vi "Main Traction Receipe Run.vi"(8 "error in (no error)":errorcluster, 11 "main ref":T1) -> (0 "error out":errorcluster)   [LabVIEW 2025]
uses:
  Traction Receipe Enum.ctl
  controls/LAB-IQ UI Data.ctl
panel:
  in  "Enum - Menu":T2
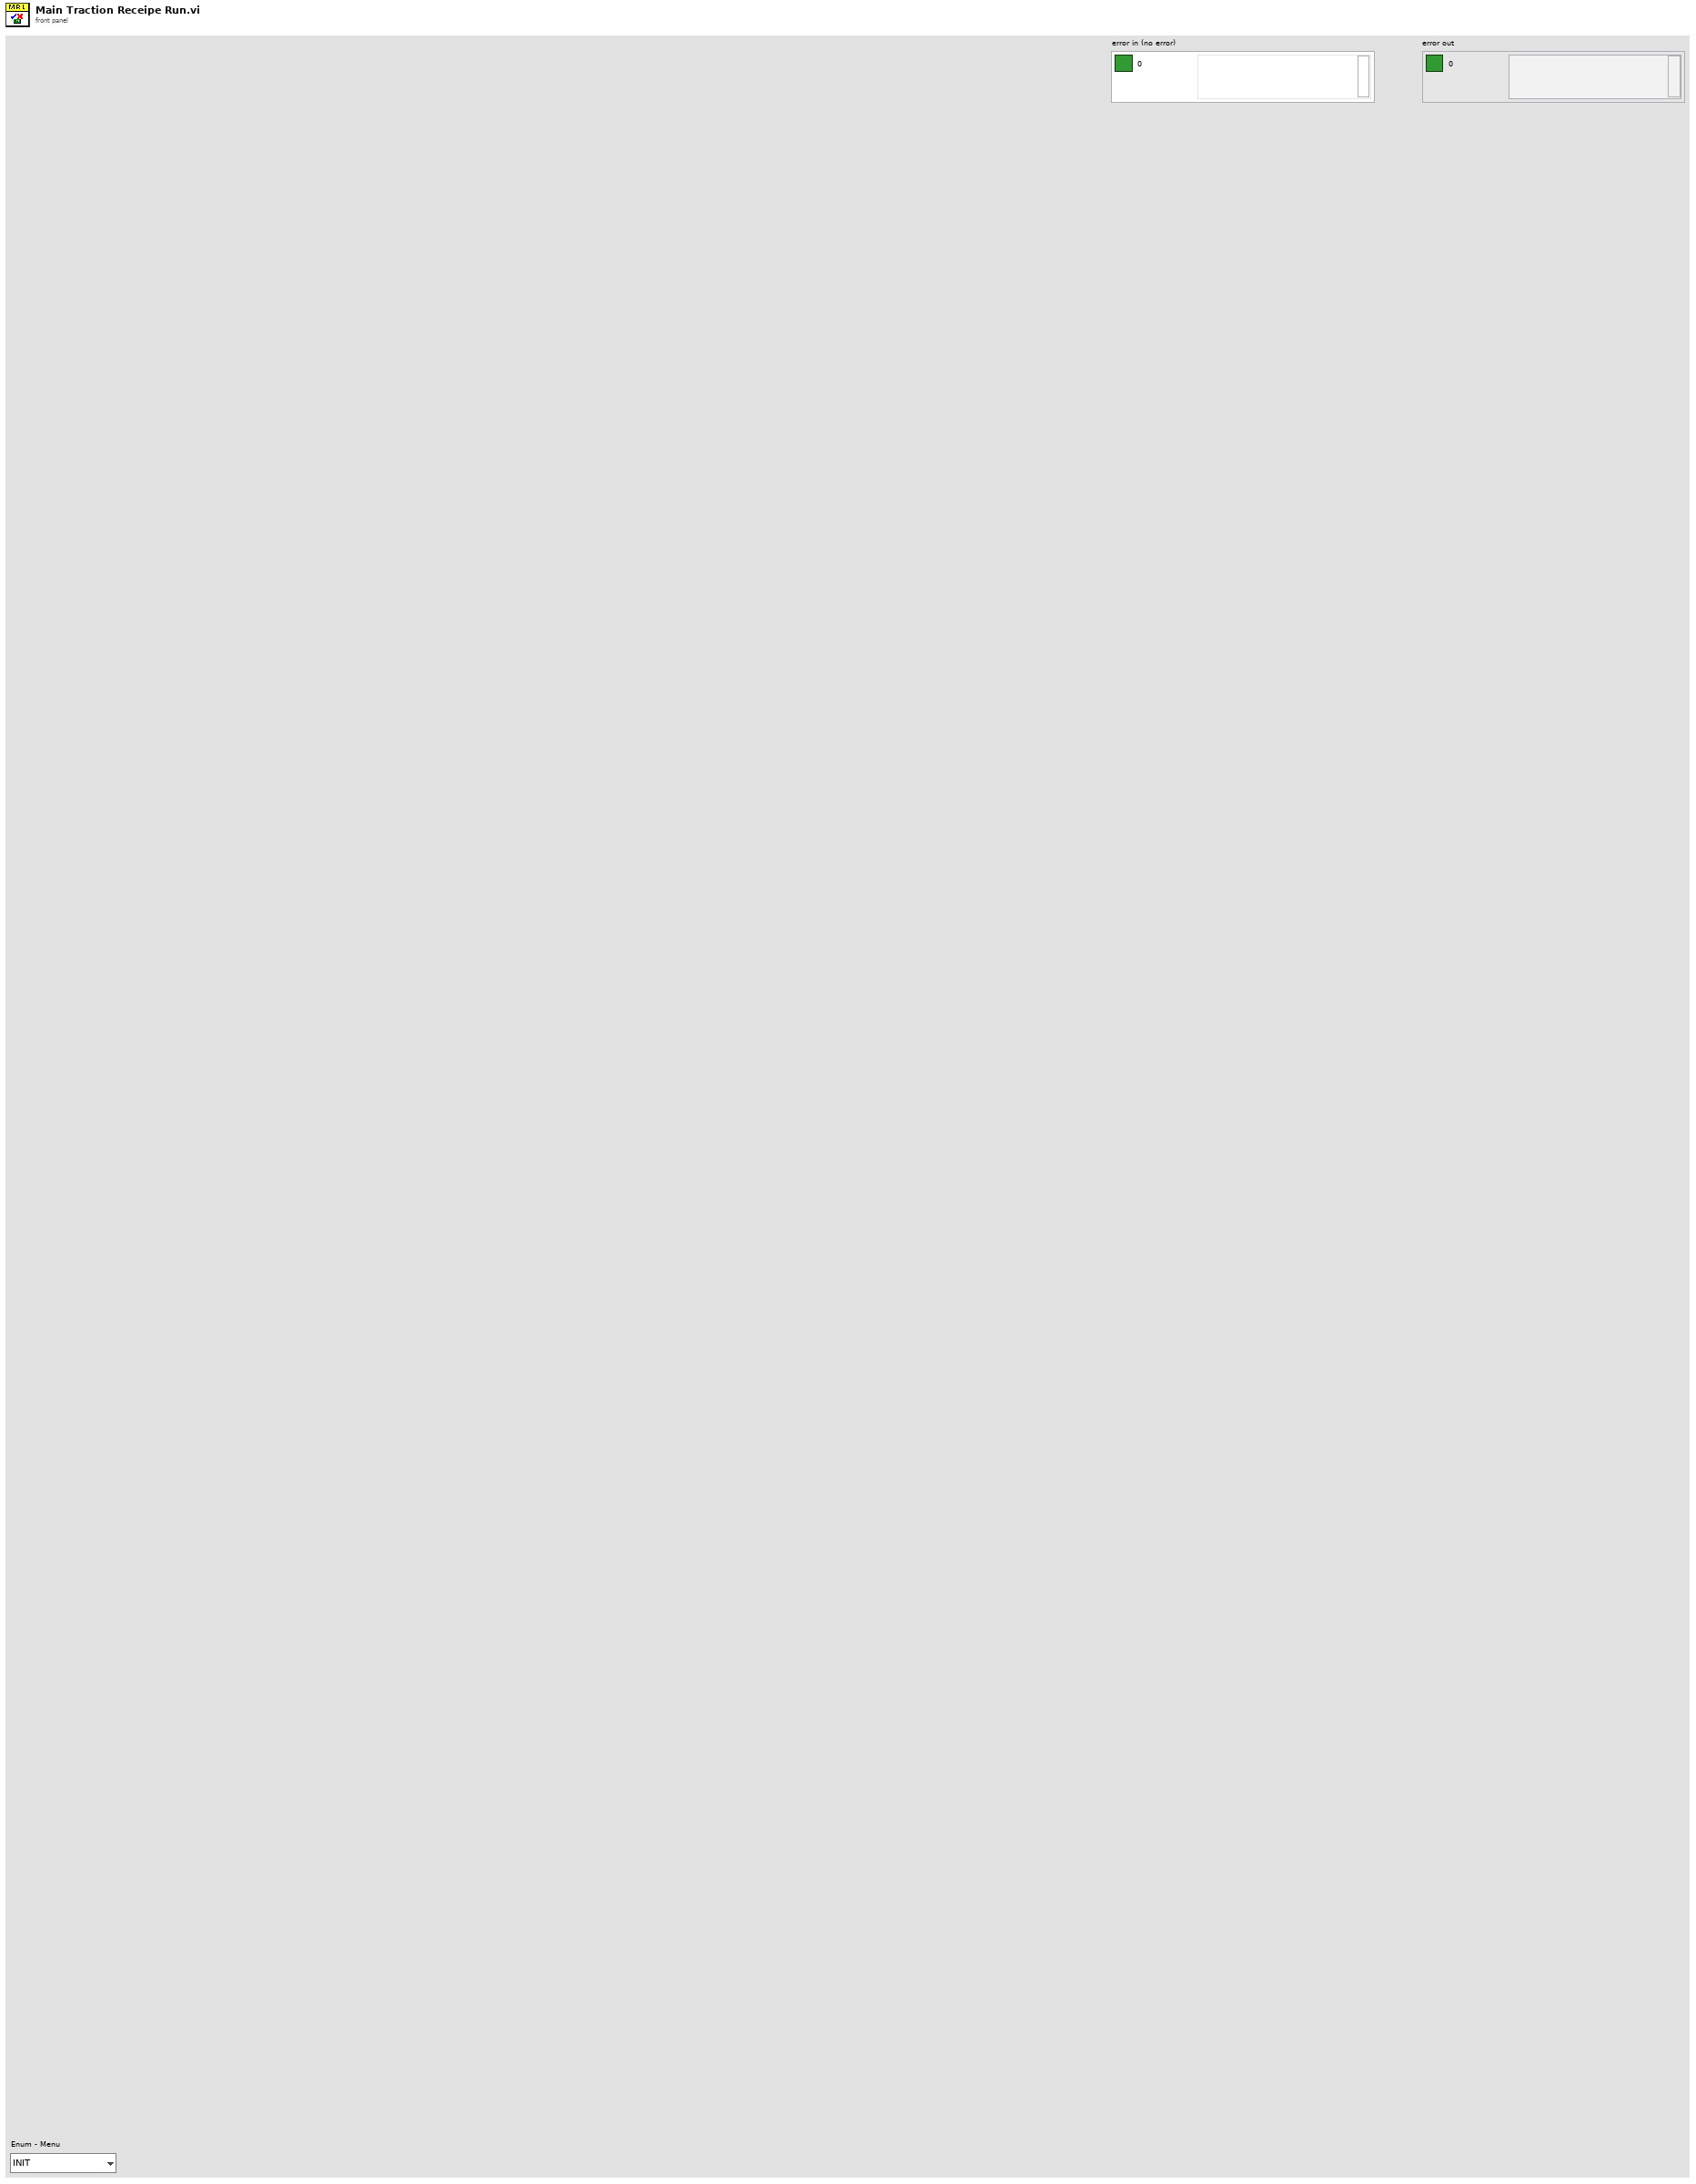
[diagram p1: front panel]
types:
  T1 = typedef "LAB-IQ UI Data.ctl" = cluster{"Main Home Screen":cluster{"GUI":refnum<vi>, "Platform Settings":refnum<vi>, "Configure":refnum<vi>, "Home":refnum<vi>, "EXIT":refnum<vi>, "service 2":refnum<vi>, "MainPage":refnum<vi>, "Analysis":refnum<vi>}, "Platform Settings":cluster{"mm/s  Surge":refnum<vi>, "Update Surge Speed":refnum<vi>, "Drive Error":refnum<vi>, "Disable Axis Jog Soft Limits":refnum<vi>, "mm/s  Sway":refnum<vi>, "Sway and Surge COM Status":refnum<vi>, "Heave COM Status":refnum<vi>, "Enable Platform":refnum<vi>, "Surge Forward Main":refnum<vi>, "Sway Right Main":refnum<vi>, "Sway Left Main":refnum<vi>, "Heave Down Main":refnum<vi>, "Heave Up main":refnum<vi>, "Update Sway Speed":refnum<vi>, "Update Heave Speed":refnum<vi>, "mm/s Heave":refnum<vi>, "mm/sec":refnum<vi>, "mm":refnum<vi>, "Surge Backward Main":refnum<vi>}, "Analysis Screen":cluster{"Analysis Home":refnum<vi>, "Surface Analysis":refnum<vi>, "Imaging":refnum<vi>, "Image Analysis":refnum<vi>, "Post Analysis":refnum<vi>}, "Config Screen":cluster{"Select Load Head":refnum<vi>, "Notes :":refnum<vi>, "FILE":refnum<vi>, "Sample ID :":refnum<vi>, "Operator ID :":refnum<vi>, "Operator Name :":refnum<vi>, "Auto":refnum<vi>}, "Motion Module":cluster{"zNL":refnum<vi>, "NL disp":refnum<vi>, "Rotary Tab":refnum<vi>, "Motion Direction:  3":refnum<vi>, "E.Velocity 2":refnum<vi>, "e.v/ssr 2":refnum<vi>, "Enter Fixed E.Velocity 2":refnum<vi>, "Enter Final SRR 2":refnum<vi>, "Enter initial SRR 2":refnum<vi>, "Enter Fixed SRR 2":refnum<vi>, "Enter the Final E.Velocity (m/s) 2":refnum<vi>, "Enter initial E.Velocity (m/s) 2":refnum<vi>, "Final Speed (RPM) 3":refnum<vi>, "Initial Speed (RPM) 2":refnum<vi>, "Enter the Final Velocity (m/s) 3":refnum<vi>, "Enter initial Velocity (m/s)  3":refnum<vi>, "Ramp Up 2":refnum<vi>, "TEST SELECTION":refnum<vi>, "SPEED SELECTION : ":refnum<vi>, "Angular Oscillation Set":refnum<vi>, "Traction":refnum<vi>, "Step Speed":refnum<vi>, "StepTable For Load-Speed":refnum<vi>, "StepTable For Speed":refnum<vi>, "Surge Forward MM":refnum<vi>, "Surge Backward MM":refnum<vi>, "M3 Image":refnum<vi>, "String 39":refnum<vi>, "Sway Left MM":refnum<vi>, "Sway Right MM":refnum<vi>, "Disable Axis Jog Soft Limits":refnum<vi>, "mm":refnum<vi>, "Heave Down MM":refnum<vi>, "Heave Up MM":refnum<vi>, "Wear Track Diameter (mm)":refnum<vi>, "Set WTD":refnum<vi>, "HomeScratch":refnum<vi>, "HomeRot":refnum<vi>, "PlaceModule":refnum<vi>, "Enter the Angle (Deg)":refnum<vi>, "Enter the Frequency (Hz)":refnum<vi>, "Motion Mode:":refnum<vi>, "LR Sway":refnum<vi>, "Rot Hor":refnum<vi>, "Scratch":refnum<vi>, "LR Cam":refnum<vi>, "MMBack":refnum<vi>, "MMNext":refnum<vi>, "Rot Ver":refnum<vi>, "Rotary Module Selection":refnum<vi>, "calculate rotary":refnum<vi>, "SPEED SELECTION : rotary":refnum<vi>, "Import 2":refnum<vi>, "Save 2":refnum<vi>, "File Path :  2":refnum<vi>, "String 45":refnum<vi>, "StepTable For Speed 3":refnum<vi>, "Enter the Speed(mm/sec)":refnum<vi>, "Enter the Speed(RPM)":refnum<vi>, "Enter Scratch Speed (mm/s):":refnum<vi>, "SwaySpeed Set":refnum<vi>, "Scartch Offset":refnum<vi>, "Motion type:":refnum<vi>, "HomeScratch 2":refnum<vi>, "Enter Scratch length (mm):":refnum<vi>, "Wear Track Diameter":refnum<vi>, "Rotary Speed Exced":refnum<vi>, "Scratch Mode":refnum<vi>, "No of Scratch":refnum<vi>}, "Environmental control":cluster{"Humidity  Status  3":refnum<vi>, "Low Temp  Status  2":refnum<vi>, "TK4 status 2":refnum<vi>, "Stage Temperature":refnum<vi>, "Sample Temperature":refnum<vi>, "Humidity (Amb)":refnum<vi>, "Clear List":refnum<vi>, "Add to list":refnum<vi>, "Wear":refnum<vi>, "Vibration":refnum<vi>, "Humidity (Chamber)":refnum<vi>, "Temperature (Chamber)":refnum<vi>, "ECR ":refnum<vi>, "Temperature (Amb)":refnum<vi>, "Microphone":refnum<vi>, "Acoustic Emission 3":refnum<vi>, "SNext":refnum<vi>, "APBack":refnum<vi>, "Enter the Temperature (°C):":refnum<vi>, "Enter the Stage \nTemperature (°C):":refnum<vi>, "Enter the Humidity (%Rh):":refnum<vi>, "Low Temp":refnum<vi>, "High Temp":refnum<vi>, "Humidity":refnum<vi>, "Sensors Picked":refnum<vi>}, "About Screen":cluster{"Password":refnum<vi>, "Home Service":refnum<vi>, "Advanced Setting":refnum<vi>, "About Tab":refnum<vi>, "ECR Port:":refnum<vi>, "Ramp Port:":refnum<vi>, "Installation/Replacement completed":refnum<vi>, "Loahead":refnum<vi>, "Heave and Surge COM Port:":refnum<vi>, "Sway COM Port:":refnum<vi>, "Temp Modbus:":refnum<vi>, "Humidity Port:":refnum<vi>, "Edit Gain Constants":refnum<vi>, "Save Gain Constants":refnum<vi>}, "Main Screen":cluster{"Main Screen Tab":refnum<vi>, "Angle and Frequency":refnum<vi>, "Stroke (mm)":refnum<vi>, "Angle (Deg)":refnum<vi>, "Main Speed Tab":refnum<vi>, "MTM MOTOR DISPLAY":refnum<vi>, "Disc Speed (m/sec)":refnum<vi>, "Ball Speed (m/sec)":refnum<vi>, "Disc Speed (RPM)":refnum<vi>, "Ball Speed (RPM)":refnum<vi>, "SPEED TAB":refnum<vi>, "Speed (m/sec)":refnum<vi>, "Set Speed (m/sec)":refnum<vi>, "Speed (RPM)":refnum<vi>, "Set Speed":refnum<vi>, "Time Tab":refnum<vi>, "Time ( HH:MM:SS ) 2":refnum<vi>, "Test Duration":refnum<vi>, "Test Duration 4":refnum<vi>, "TEST CYCLE":refnum<vi>, "TOTAL CYCLES":refnum<vi>, "Set Load (N)":refnum<vi>, "Temp Tabs":refnum<vi>, "Heater":refnum<vi>, "TK4 status":refnum<vi>, "ChamberTemp":refnum<vi>, "SetTmp":refnum<vi>, "Controller  Status":refnum<vi>, "ChamberTemp 2":refnum<vi>, "SetTmp 2":refnum<vi>, "Controller  Status 2":refnum<vi>, "ChamberTemp 3":refnum<vi>, "SetTmp 3":refnum<vi>, "Cooling":refnum<vi>, "Load Communication":refnum<vi>, "Ambient \nTemperature":refnum<vi>, "HumCOMStatus":refnum<vi>, "Ambient\n Humidity":refnum<vi>, "Freq (Hz)":refnum<vi>, "Load En":refnum<vi>, "NLt":refnum<vi>, "zNL 2":refnum<vi>, "Humidity On":refnum<vi>, "humidity disp":refnum<vi>, "Set Humidity":refnum<vi>, "NL disp 2":refnum<vi>, "Humidity On 2":refnum<vi>, "humidity disp 2":refnum<vi>, "Set Humidity 2":refnum<vi>, "NL disp 3":refnum<vi>, "AppLoadSeq scratch":refnum<vi>, "Stop Scratch":refnum<vi>, "ClrLog":refnum<vi>, "Trip Log":refnum<vi>, "STOP":refnum<vi>, "Start Test":refnum<vi>, "Test status":refnum<vi>, "AR Led":refnum<vi>, "Data":refnum<vi>, "Health":refnum<vi>, "Sway COM Status":refnum<vi>, "Heave COM Status":refnum<vi>, "Grp Tab":refnum<vi>, "Sub Graph":refnum<vi>, "SD (mm)":refnum<vi>, "Siliding distance Reset Graph":refnum<vi>, "SDGp":refnum<vi>, "Humidity Reset Graph":refnum<vi>, "HumrGp":refnum<vi>, "Acoustic Emission (mV)":refnum<vi>, "Aqucostic Reset Graph":refnum<vi>, "gACQUOS":refnum<vi>, "ECR RESET":refnum<vi>, "ECR":refnum<vi>, "Temperature Reset":refnum<vi>, "Acoustic Emission (mV) 2":refnum<vi>, "Aqucostic Reset Graph 2":refnum<vi>, "gACQUOS 2":refnum<vi>, "ECR RESET 2":refnum<vi>, "ECR 2":refnum<vi>, "Temperature Reset 2":refnum<vi>, "Temperature (deg c)":refnum<vi>, "Speed Reset Graph":refnum<vi>, "Speed Tab":refnum<vi>, "MTM DISC  SPEED":refnum<vi>, "MTM BALL SPEED":refnum<vi>, "speed mm/sec":refnum<vi>, "Hymidity":refnum<vi>, "Humidity Disable trip":refnum<vi>, "CoF Trip  2":refnum<vi>, "Depth Trip":refnum<vi>, "Weart Deapth":refnum<vi>, "Depth Reset Graph":refnum<vi>, "Weart":refnum<vi>, "Depthz":refnum<vi>, "Depth (µm)":refnum<vi>, "WearGp":refnum<vi>, "NL Trip 2":refnum<vi>, "Load pid":refnum<vi>, "Load Disable Trip":refnum<vi>, "Load Reset Graph":refnum<vi>, "NL Display 4":refnum<vi>, "Main Chart 3":refnum<vi>, "BACK":refnum<vi>, "Depth Trip 2":refnum<vi>, "COF TRIP ":refnum<vi>, "Friction Force (N)":refnum<vi>, "FF Reset Graph":refnum<vi>, "FF Disable Trip":refnum<vi>, "FF TRIP":refnum<vi>, "COF Disable Trip":refnum<vi>, "COF Reset Graph":refnum<vi>, "Start Test Temp":refnum<vi>, "zFF":refnum<vi>, "Friction Force (N) Graph":refnum<vi>, "Coefficient of Friction":refnum<vi>, "Scratch Start Test":refnum<vi>, "FF Tab":refnum<vi>, "Cyclic Friction Force (N)":refnum<vi>, "CZ FF":refnum<vi>, "Cyclic Friction Force (N) Graph":refnum<vi>, "Cyclic Coefficient of Friction":refnum<vi>, "Cyclic FF TRIP":refnum<vi>, "Cyclic FF Disable Trip":refnum<vi>, "cyclic COF Disable Trip":refnum<vi>, "cyclic COF TRIP":refnum<vi>, "cyclic COF Reset Graph":refnum<vi>, "Cyclic FF Reset Graph":refnum<vi>, "Test Trip":refnum<vi>, "Multi Scratch Pass":refnum<vi>, "Scratch Start Recording":refnum<vi>}, "Loading":cluster{"Indentation":refnum<vi>, "Reference Sample":refnum<vi>, "Load Cell Communication Slide":refnum<vi>, "com 3":refnum<vi>, "com":refnum<vi>, "DecaForce COM Status":refnum<vi>, "Update":refnum<vi>, "Clear 3":refnum<vi>, "seq":refnum<vi>, "Stribeck table":refnum<vi>, "Stribeck Table  For loading":refnum<vi>, "Loading Mode":refnum<vi>, "Enter the Final Load (N)":refnum<vi>, "Enter the CoF Trip":refnum<vi>, "Enter the Friction Force Trip":refnum<vi>, "Enter the Normal load Trip":refnum<vi>, "Enter the Load  (N)":refnum<vi>, "KiloForce":refnum<vi>, "DecaForce ":refnum<vi>, "MicroForce":refnum<vi>, "LHBack":refnum<vi>, "LHNext":refnum<vi>, "Enter the Loading Rate (N/min)":refnum<vi>, "Message":refnum<vi>, "Warning 2":refnum<vi>, "SSP 0.75":refnum<vi>, "SSP 0.5":refnum<vi>, "SSP 0.3":refnum<vi>, "Warning":refnum<vi>, "gui GIF":refnum<vi>, "Communication is established":refnum<vi>, "AppLoad 4":refnum<vi>, "Multipoint":refnum<vi>, "Load Selection":refnum<vi>}, "PID":cluster{"Ramp MulFac":refnum<vi>, "pulses LoadDiffRamp(2..10)":refnum<vi>, "PulseControlRamp(diff<=3N)":refnum<vi>, "SetLoadDeadband(%) Load(0-10N)":refnum<vi>, "PID gains out delay (microForce)":refnum<vi>, "Ramp":refnum<vi>, "Gain 2":refnum<vi>, "pulses LoadDiff(2..10)":refnum<vi>, "pulses LoadDiff(11..50)":refnum<vi>, "PulseControl(diff<=3N)":refnum<vi>, "SetLoadDeadband(%)  2":refnum<vi>, "Dummy Run":refnum<vi>, "Vertical load (N)":refnum<vi>, "AutoTune":refnum<vi>, "Offset 3 ":refnum<vi>, "apply load":refnum<vi>, "Offset  3":refnum<vi>, "apply load 2":refnum<vi>, "Enter ByPass Load":refnum<vi>, "reinit 3":refnum<vi>, "output range delay":refnum<vi>, "PID gains out delay":refnum<vi>, "Bypass Load":refnum<vi>, "pulsesSent":refnum<vi>, "pulses ":refnum<vi>, "actpid":refnum<vi>, "gFF Rot":refnum<vi>, "pulses LoadDiff(21..1000)":refnum<vi>, "Delay":refnum<vi>, "deadband":refnum<vi>}, "Config Parameters":cluster{"Tab Control 3":refnum<vi>, "Tab Control 19":refnum<vi>, "SAMPLES":refnum<vi>, "Re-initilaize":refnum<vi>, "Filter ON/OFF":refnum<vi>, "TracHomeSurgeOffsetCounts 10MM":refnum<vi>, "TracHomeSwayOffsetCounts 10MM":refnum<vi>, "Acoustic Emission:":refnum<vi>, "Apply Filter (FF)":refnum<vi>, "Filter% 2":refnum<vi>, "Apply Filter (Load)":refnum<vi>, "Filter% ":refnum<vi>, "Sway distance (mm)":refnum<vi>, "Surge distance (mm)":refnum<vi>, "DataSavingLoopDelay(ms)":refnum<vi>, "SAVE 2":refnum<vi>, "Enter Distance":refnum<vi>, "Sway Counts:":refnum<vi>, "Distance (mm): 3":refnum<vi>, "Surge Counts:":refnum<vi>, "Distance (mm): 2":refnum<vi>, "Distance (mm):":refnum<vi>, "Heave Counts:":refnum<vi>, "LRMHomeSurgeOffsetCounts":refnum<vi>, "LRMHomeSwayOffsetCounts":refnum<vi>, "TracHomeSurgeOffsetCounts 20MM":refnum<vi>, "TracHomeSwayOffsetCounts 20MM":refnum<vi>, "RotHomeSwayOffsetCounts":refnum<vi>, "RotHomeSurgeOffsetCounts":refnum<vi>, "Heave distance":refnum<vi>, "Zmm":refnum<vi>, "Heave Pulses/mm":refnum<vi>, "Surge Pulses/mm":refnum<vi>, "Sway Pulses/mm":refnum<vi>, "Heave Pitch":refnum<vi>, "Surge Pitch":refnum<vi>, "Sway Pitch":refnum<vi>, "Heave PPR":refnum<vi>, "Surge PPR":refnum<vi>, "Sway PPR":refnum<vi>, "Tab Control 5":refnum<vi>, "Tab Control 14":refnum<vi>, "Tab Control 26":refnum<vi>, "AE":refnum<vi>, "Heave Loop Delay":refnum<vi>, "Heave PID Speed":refnum<vi>, "Surge Jog Speed":refnum<vi>, "Heave Jog Speed":refnum<vi>, "Sway Loop Delay":refnum<vi>, "Sway PID Speed":refnum<vi>, "Sway Jog Speed":refnum<vi>, "DEPTH TRIP VALUE":refnum<vi>, "LOAD TRIP VALUE":refnum<vi>, "DEPTH TRIP   ENABLE":refnum<vi>, "LOAD TRIP  ENABLE":refnum<vi>, "CYCLIC FF TRIP VALUE":refnum<vi>, "FF TRIP VALUE":refnum<vi>, "CYCLIC CoF TRIP VALUE":refnum<vi>, "COF TRIP VALUE":refnum<vi>, "CYCLIC COF TRIP  ENABLE":refnum<vi>, "CYCLIC FF TRIP  ENABLE":refnum<vi>, "FF TRIP  ENABLE":refnum<vi>, "COF TRIP  ENABLE":refnum<vi>, "JOG TRIP LOAD VALUE (N)":refnum<vi>, "Rotary Vertical":refnum<vi>, "Traction":refnum<vi>, "Scratch":refnum<vi>, "LRM CAM":refnum<vi>, "Sway LRM":refnum<vi>, "Rotary Horizontal":refnum<vi>}, "Loading Com Port":cluster{"ClearAll":refnum<vi>, "Mz(Nm)":refnum<vi>, "My(Nm)":refnum<vi>, "Mx(Nm)":refnum<vi>, "Save Dwell":refnum<vi>, "Acq Delay (ms)":refnum<vi>, "Burst Delay (ms)":refnum<vi>, "model":refnum<vi>, "SN":refnum<vi>, "FFx(N)":refnum<vi>, "Sensor IP":refnum<vi>, "Port":refnum<vi>, "FFy(N)":refnum<vi>, "Load(N)":refnum<vi>, "delete Handle":refnum<vi>, "Create Handle":refnum<vi>, "ft_data":refnum<vi>, "ft_range":refnum<vi>, "ft_data 2":refnum<vi>, "stop 6":refnum<vi>, "running_flag":refnum<vi>, "ft_udp_handle":refnum<vi>, "get-data-return":refnum<vi>, "get-range-return":refnum<vi>, "zero-return":refnum<vi>, "filter-return":refnum<vi>, "initial-return":refnum<vi>, "deleteHandle-result":refnum<vi>, "Load Cell Temp":refnum<vi>, "Load Cell":refnum<vi>, "ZeroAll":refnum<vi>, "FORCE (N)":refnum<vi>, "TORQUE (N-m)":refnum<vi>}, "Heave AND Surge":cluster{"SURGE POSE":refnum<vi>, "error out Read":refnum<vi>, "HEAVE POSE":refnum<vi>, "State":refnum<vi>, "Homed":refnum<vi>, "Sequence ID":refnum<vi>, "error out Write":refnum<vi>, "faultCode":refnum<vi>, "Ack ID":refnum<vi>, "SPEED":refnum<vi>, "Distance":refnum<vi>, "Mode Command":refnum<vi>, "Heave and Surge Read":refnum<vi>, "Read Heave Temp":refnum<vi>, "Spare 15":refnum<vi>, "Spare 14":refnum<vi>, "Spare 13":refnum<vi>, "Spare 12":refnum<vi>, "Spare 11":refnum<vi>, "Spare 10":refnum<vi>, "Spare 9":refnum<vi>, "Spare 8":refnum<vi>, "Spare 7":refnum<vi>, "Spare 6":refnum<vi>, "Spare 5":refnum<vi>, "Spare 4":refnum<vi>, "Spare 2":refnum<vi>, "Spare 1":refnum<vi>, "Node Id":refnum<vi>, "Spare 3":refnum<vi>, "SPARE 4":refnum<vi>, "SPARE 3":refnum<vi>, "SPARE 2":refnum<vi>, "SPARE 1":refnum<vi>, "fwMajor":refnum<vi>, "fwMinor":refnum<vi>, "Manual Write":refnum<vi>, "Heave and Surge Write":refnum<vi>, "SPARE 5":refnum<vi>, "Reserved ":refnum<vi>, "SPARE 8":refnum<vi>, "SPARE 6":refnum<vi>, "SPARE 7":refnum<vi>, "SPARE 17":refnum<vi>, "SPARE 16":refnum<vi>, "SPARE 15":refnum<vi>, "SPARE 14":refnum<vi>, "SPARE 13":refnum<vi>, "SPARE 12":refnum<vi>, "SPARE 11":refnum<vi>, "SPARE 10":refnum<vi>, "SPARE 9":refnum<vi>, "System UPTIME":refnum<vi>, "Missed Packets":refnum<vi>, "faultCode Surge Right":refnum<vi>, "faultCode Surge Left":refnum<vi>, "faultCode Heave":refnum<vi>, "UPLINK HEAVE":refnum<vi>, "DOWNLINK HEAVE":refnum<vi>}, "New PID LOGIC":cluster{"Fine Tune Zone":refnum<vi>, "PID SDelay":refnum<vi>, "Max_pos_limit":refnum<vi>, "Min_pos_limit":refnum<vi>, "i_limit":refnum<vi>, "pct_scale":refnum<vi>, "Deadband":refnum<vi>, "Kd":refnum<vi>, "Ki":refnum<vi>, "Kp":refnum<vi>, "Current Position":refnum<vi>, "Set Load":refnum<vi>, "Current Load":refnum<vi>, "Pulse delta":refnum<vi>, "Init Step":refnum<vi>, "Max Step Linit":refnum<vi>, "min_deadband_floor":refnum<vi>, "dynamic_spindle_noise_scalar":refnum<vi>, "min_finetune_floor":refnum<vi>, "filter_alpha":refnum<vi>, "PID":refnum<vi>}, "SWAY ":cluster{"fwMajor":refnum<vi>, "Homed":refnum<vi>, "Rotary POSE":refnum<vi>, "State":refnum<vi>, "SWAY POSE":refnum<vi>, "Ack ID":refnum<vi>, "faultCode":refnum<vi>, "Node Id":refnum<vi>, "fwMinor":refnum<vi>, "Spare 6":refnum<vi>, "Spare 5":refnum<vi>, "Spare 4":refnum<vi>, "Spare 3":refnum<vi>, "Spare 2":refnum<vi>, "Spare 1":refnum<vi>, "Spare 7":refnum<vi>, "SPARE  5":refnum<vi>, "error out Write  SWAY ":refnum<vi>, "error out Read SWAY ":refnum<vi>, "Manual Write SWAY ":refnum<vi>, "SWAY WRITE":refnum<vi>, "SPARE  4":refnum<vi>, "SPARE  3":refnum<vi>, "SPARE 2":refnum<vi>, "SPARE 1":refnum<vi>, "Spare 15":refnum<vi>, "Spare 14":refnum<vi>, "Spare 13":refnum<vi>, "Spare 12":refnum<vi>, "Spare 11":refnum<vi>, "Spare 9":refnum<vi>, "Spare 8":refnum<vi>, "SPEED":refnum<vi>, "Distance":refnum<vi>, "Mode Command":refnum<vi>, "Sequence ID":refnum<vi>, "SWAY READ":refnum<vi>, "Spare 10":refnum<vi>, "Read SWAY Temp":refnum<vi>, "faultCode Sway ":refnum<vi>, "Missed Packets":refnum<vi>, "System UPTIME sway":refnum<vi>, "SPARE 6":refnum<vi>, "SPARE 7":refnum<vi>, "SPARE 9":refnum<vi>, "SPARE 11":refnum<vi>, "SPARE 10":refnum<vi>, "SPARE 8":refnum<vi>, "SPARE 13":refnum<vi>, "SPARE 12":refnum<vi>, "SPARE 17":refnum<vi>, "SPARE 16":refnum<vi>, "SPARE 15":refnum<vi>, "SPARE 14":refnum<vi>, "Reserved":refnum<vi>, "faultCode Rotary":refnum<vi>, "UPLINK SWAY":refnum<vi>, "DOWNLINK SWAY":refnum<vi>}, "Analysis Screen":cluster{"Analysis Home":refnum<vi>, "Refresh 2":refnum<vi>, "MEAN 4":refnum<vi>, "SD 4":refnum<vi>, "VARIANCE 4":refnum<vi>, "MEAN  3":refnum<vi>, "SD  3":refnum<vi>, "VARIANCE  3":refnum<vi>, "MEAN 2":refnum<vi>, "SD  2":refnum<vi>, "VARIANCE 2":refnum<vi>, "MEAN":refnum<vi>, "SD":refnum<vi>, "VARIANCE":refnum<vi>, "File 4 Discription":refnum<vi>, "OPEN 4":refnum<vi>, "File Name 4":refnum<vi>, "OPEN 3":refnum<vi>, "File 3 Discription":refnum<vi>, "File Name 3":refnum<vi>, "Y-AXIS":refnum<vi>, "X-AXIS":refnum<vi>, "XY Graph":refnum<vi>, "File Name 2":refnum<vi>, "File Name 1":refnum<vi>, "OPEN 2":refnum<vi>, "OPEN 1":refnum<vi>, "File 1 Discription ":refnum<vi>, "File 2 Discription":refnum<vi>, "Export":refnum<vi>, "File Format":refnum<vi>}, "Traction":cluster{"faultCode Traction 2":refnum<vi>, "faultCode Traction 1":refnum<vi>, "Missed Packets":refnum<vi>, "System UPTIME Traction":refnum<vi>, "SPARE 17":refnum<vi>, "SPARE 16":refnum<vi>, "SPARE 15":refnum<vi>, "SPARE 14":refnum<vi>, "SPARE 13":refnum<vi>, "SPARE 12":refnum<vi>, "SPARE 11":refnum<vi>, "SPARE 10":refnum<vi>, "SPARE 9":refnum<vi>, "SPARE 8":refnum<vi>, "SPARE 7":refnum<vi>, "SPARE 6":refnum<vi>, "Reserved":refnum<vi>, "SPARE  5":refnum<vi>, "Manual Write TRACTION":refnum<vi>, "TRACTION WRITE":refnum<vi>, "SPARE  4":refnum<vi>, "SPARE  3":refnum<vi>, "SPARE 2":refnum<vi>, "SPARE 1":refnum<vi>, "Spare 7":refnum<vi>, "Spare 6":refnum<vi>, "Spare 5":refnum<vi>, "Spare 4":refnum<vi>, "Spare 2":refnum<vi>, "Spare 1":refnum<vi>, "Node Id":refnum<vi>, "Read TRACTION Temp":refnum<vi>, "fwMinor":refnum<vi>, "fwMajor":refnum<vi>, "faultCode":refnum<vi>, "TRACTION POSE":refnum<vi>, "TRACTION POSE 2":refnum<vi>, "Homed":refnum<vi>, "State":refnum<vi>, "Ack ID":refnum<vi>, "SPEED":refnum<vi>, "Distance":refnum<vi>, "Mode Command":refnum<vi>, "Sequence ID":refnum<vi>, "error out Read TRACTION":refnum<vi>, "error out Write  TRACTION":refnum<vi>, "TRACTION READ":refnum<vi>, "Spare 3":refnum<vi>, "Downlink traction":refnum<vi>, "Uplink Traction":refnum<vi>}, "Traction reciepe":cluster{"SRR Sweep Range (%) Stribeck":refnum<vi>, "Traction Receipe":refnum<vi>, "Total Execution Time":refnum<vi>, "Total Steps":refnum<vi>, "Duration / Step (s)  Stribeck":refnum<vi>, "STRIBECK Fixed SRR List (%)":refnum<vi>, "Duration / Step (s) Traction":refnum<vi>, "SRR Sweep Range (%) traction":refnum<vi>, "Rolling Speed (mm/s)":refnum<vi>, "Temperature Stages (°C)":refnum<vi>, "Ball Load (N)":refnum<vi>, "Lubricant Name":refnum<vi>, "Profile File Name":refnum<vi>, "SET entrainment Velocity":refnum<vi>, "Test Array Size":refnum<vi>, "SRR INDEX [ STRIBECK]":refnum<vi>, "Stribeck Size":refnum<vi>, "SET SRR":refnum<vi>, "ELAPSED TIMER ":refnum<vi>, "BALL SET RPM":refnum<vi>, "DISC SET RPM":refnum<vi>, "SET LOAD":refnum<vi>, "TEMPERATURE READ":refnum<vi>, "SET TEMPERATURE":refnum<vi>, "Traction Size":refnum<vi>, "DISC SPEED (rpm)":refnum<vi>, "BALL SPEED (rpm)":refnum<vi>, "BALL WEAR TRACK":refnum<vi>, "DISC WEARTRACK":refnum<vi>, "SRR INDEX [ TRACTION]":refnum<vi>, "Start Index Type":refnum<vi>, "Enum - Menu":refnum<vi>, "Ball (mm/sec)":refnum<vi>, "Disc (mm/sec)":refnum<vi>}, "Traction Control":cluster{"HomeTraction":refnum<vi>, "Demo Mode Display":refnum<vi>, "Traction Message":refnum<vi>, "Traction Step Update Details":refnum<vi>, "Main Tab sequence for selection":refnum<vi>, "Ramp Tab":refnum<vi>, "e.v/ssr":refnum<vi>, "Enter Fixed E.Velocity":refnum<vi>, "Enter Final SRR":refnum<vi>, "Enter initial SRR":refnum<vi>, "Enter Fixed SRR":refnum<vi>, "Enter the Final E.Velocity (m/s)":refnum<vi>, "Enter initial E.Velocity (m/s)":refnum<vi>, "Ball WTD":refnum<vi>, "E.Velocity":refnum<vi>, "Enter the Final Velocity (m/s)":refnum<vi>, "Enter initial Velocity (m/s)":refnum<vi>, "Ramp Up   Disc":refnum<vi>, "Initial DiscSpeed (RPM)":refnum<vi>, "Final Speed (RPM) Ball":refnum<vi>, "Final Speed (RPM)":refnum<vi>, "Initial Speed (RPM) Ball":refnum<vi>, "Enter the Final Velocity (m/s) Ball":refnum<vi>, "Enter initial Velocity (m/s) Ball":refnum<vi>, "Ramp Up":refnum<vi>, "ExceedBallSpeed step":refnum<vi>, "ExceedDiscSpeed":refnum<vi>, "BallSpeed Exceed Indication":refnum<vi>, "Apply":refnum<vi>, "SPEED SELECTION : MTM":refnum<vi>, "SPEED SELECTION : MTM 2":refnum<vi>, "TEST SELECTION (MTM)":refnum<vi>, "MTM Test Selection":refnum<vi>, "File Path Tab":refnum<vi>, "File Path String":refnum<vi>, "Save":refnum<vi>, "Save  2":refnum<vi>, "Import ":refnum<vi>, "File Path :":refnum<vi>, "Step Sequence Indication Tab":refnum<vi>, "Step Sequence Indication":refnum<vi>, "Calculate Step":refnum<vi>, "StepTable":refnum<vi>, "ExceedDiscSpeed  Cinstant Speed":refnum<vi>, "ExceedBallSpeed Constant":refnum<vi>, "TEST SELECTION (MTM) 2":refnum<vi>, "SPEED SELECTION : MTM 3":refnum<vi>, "MTM Test Selection 2":refnum<vi>, "Enter the Speed (m/sec): ":refnum<vi>, "Enter the Speed (m/sec):  2":refnum<vi>, "Enter the Speed (RPM):":refnum<vi>, "Lower Spped ":refnum<vi>, "Upper":refnum<vi>, "Enter the Speed (RPM):Ball":refnum<vi>, "Disc Motion Direction: ":refnum<vi>, "Ball Motion Direction :":refnum<vi>, "Motion Mode: ":refnum<vi>, "Wear Track Diameter (mm) ":refnum<vi>, "Disc Speed Indicator":refnum<vi>, "ExceedBallSpeed":refnum<vi>}, "Acquostic":cluster{"Last Config Rejected ":refnum<vi>, "rx command count":refnum<vi>, "Current Filter Id":refnum<vi>, "Isolated Gain":refnum<vi>, "DAQ Status":refnum<vi>, "error out":refnum<vi>, "error in (no error)":refnum<vi>, "Uplink Packet":refnum<vi>, "data out":refnum<vi>, "Downlink Packet":refnum<vi>, "Signal Energy":refnum<vi>, "Amplitude db_AE":refnum<vi>, "Peak Amplitude":refnum<vi>, "AE Ring-Down Counts":refnum<vi>, "Gains":refnum<vi>, "Manual Write Acquostic":refnum<vi>}}
  T2 = typedef "Traction Receipe Enum.ctl" = enum16{"INIT", "START", "TRACTION", "STRIBECK", "MAIN INDEX INCREMENT", "TEMPERATURE SET", "TEMPERATURE REACH", "CHURNING START", "CHURNING STOP", "LOAD", "LOAD REACHED", "SRR SET", "SRR WAIT", "SRR INCREMENT", "SPEED SET", "SPEED WAIT", "SPEED INCREMENT", "UNLOAD", "CLOSE"}
  T3 = enum8{"Enabled", "Disabled", "Disabled and Grayed Out"}
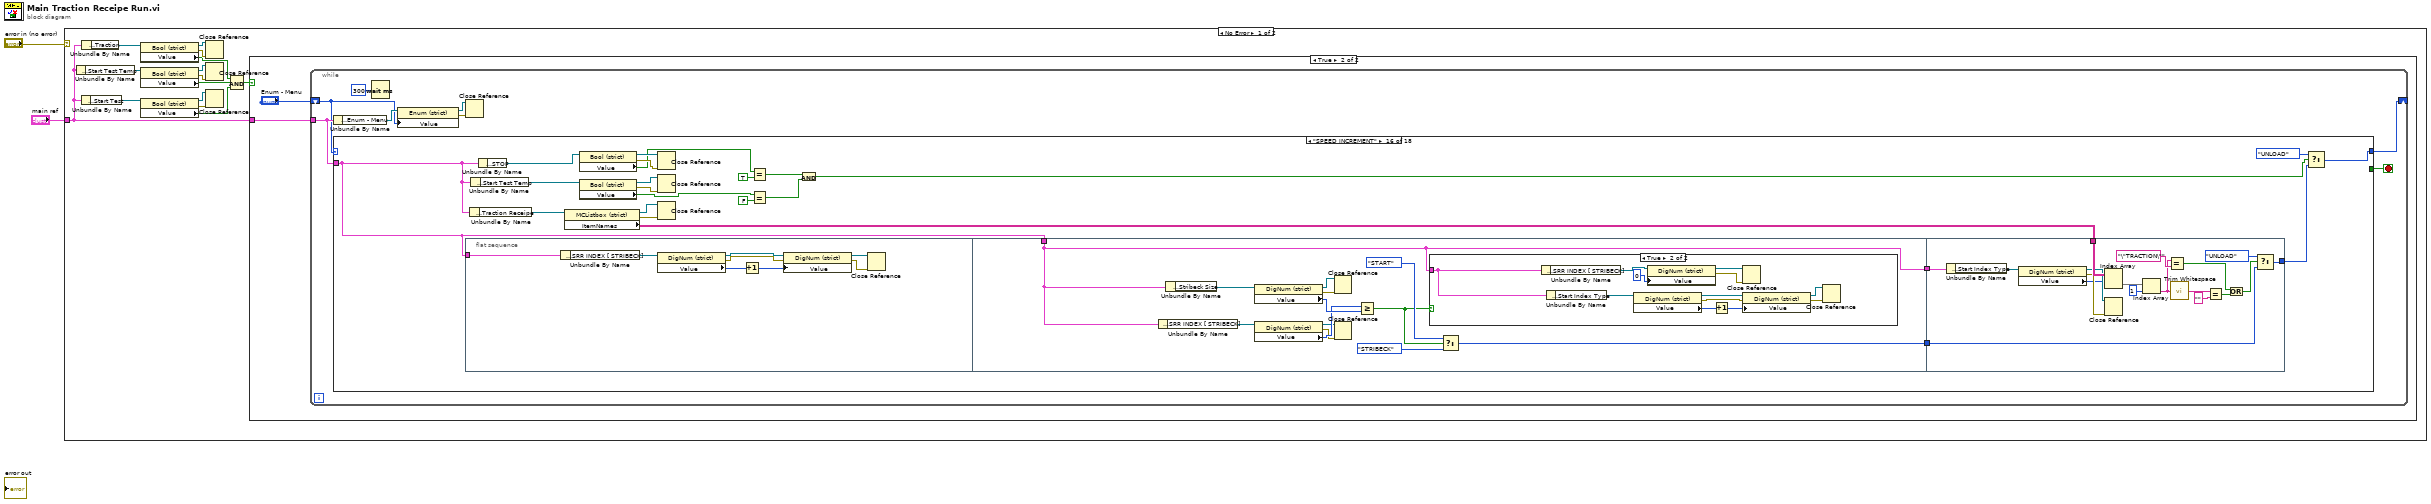
[diagram p0: block diagram]
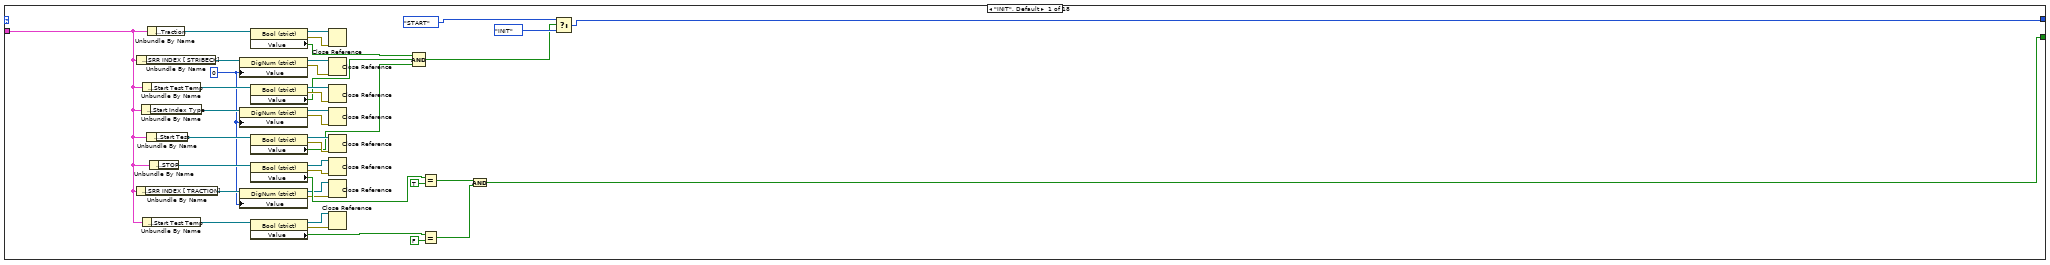
[diagram p3: hidden frame]
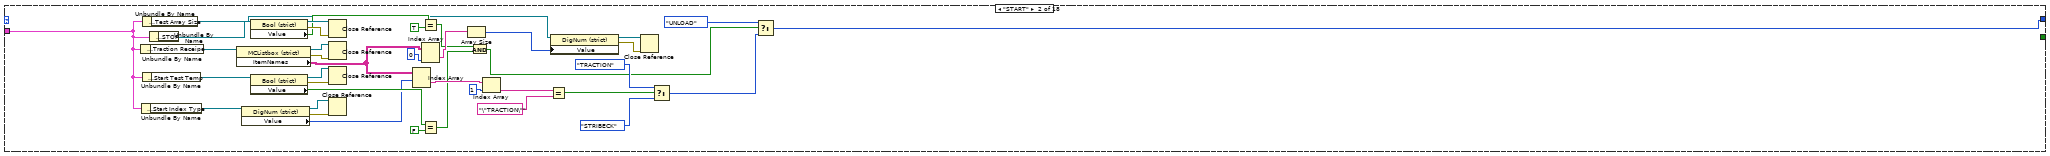
[diagram p4: hidden frame]
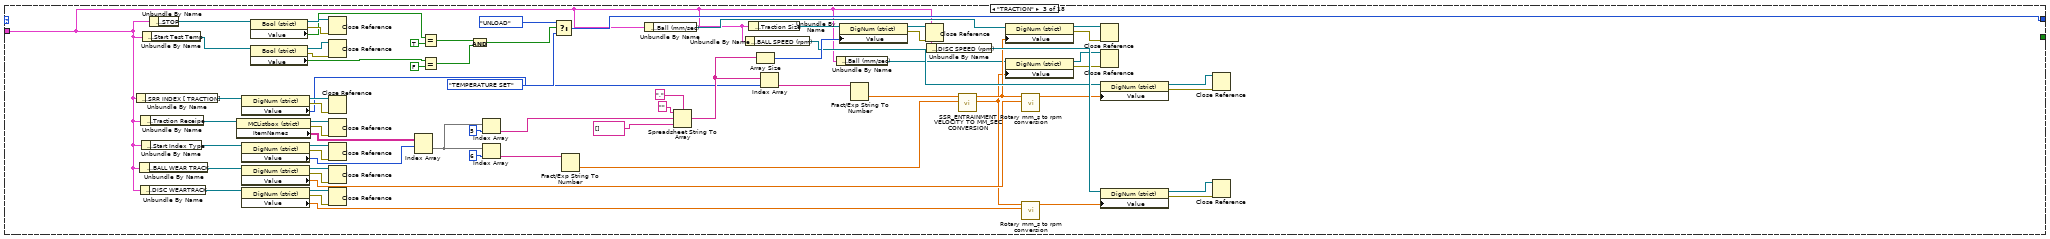
[diagram p5: hidden frame]
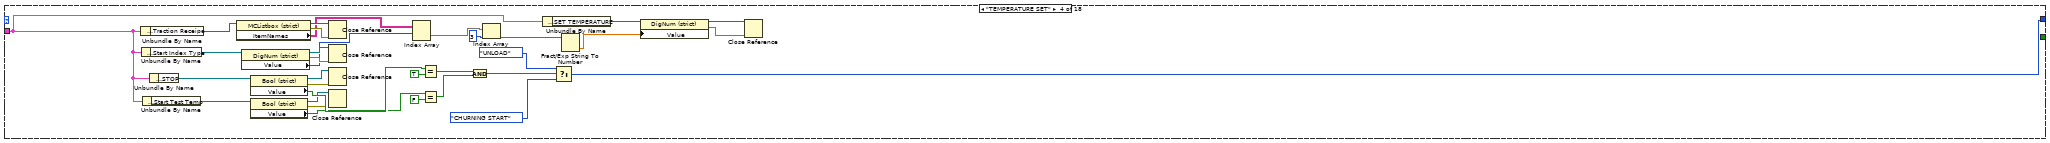
[diagram p6: hidden frame]
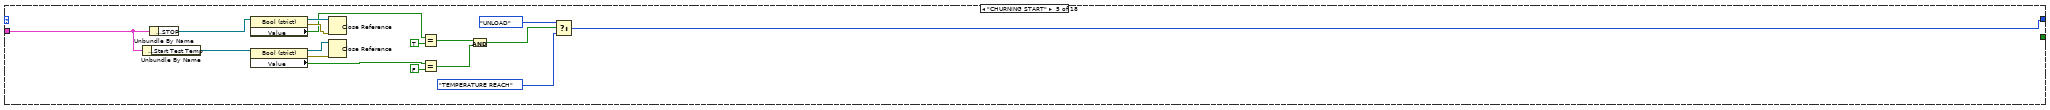
[diagram p7: hidden frame]
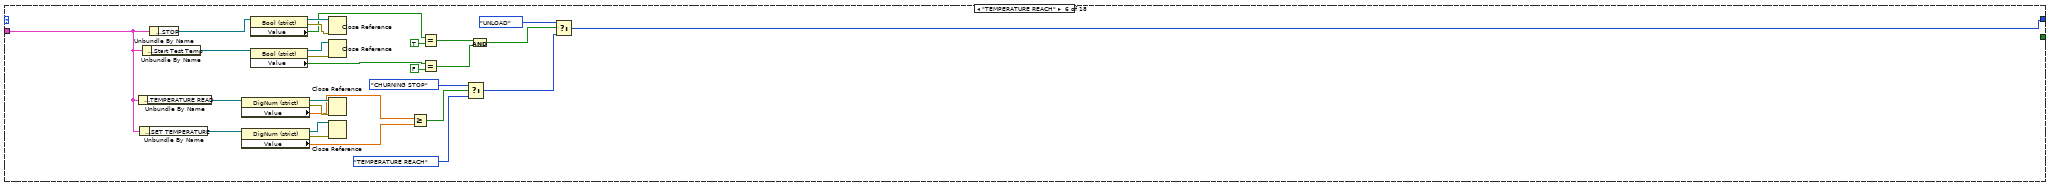
[diagram p8: hidden frame]
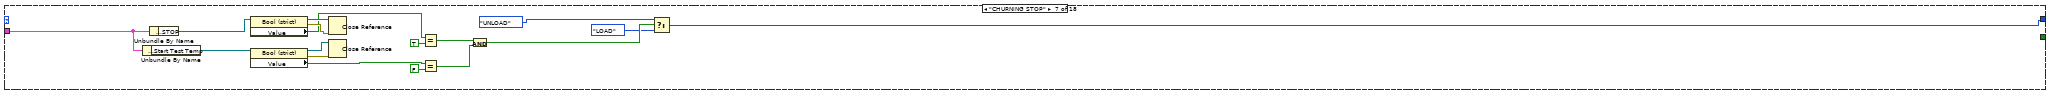
[diagram p9: hidden frame]
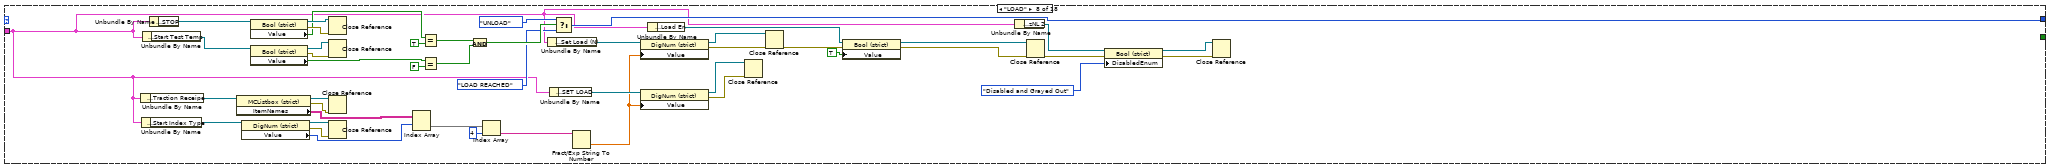
[diagram p10: hidden frame]
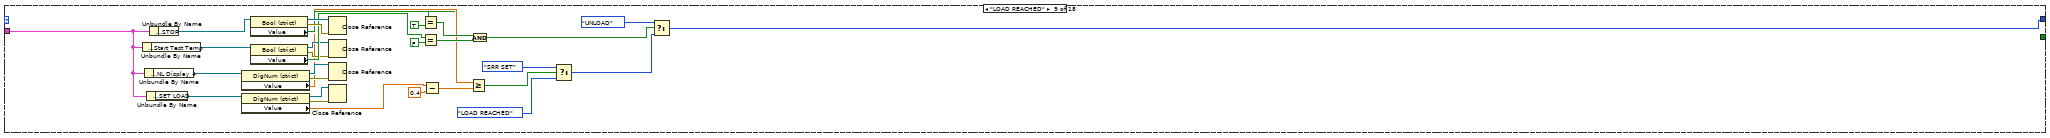
[diagram p11: hidden frame]
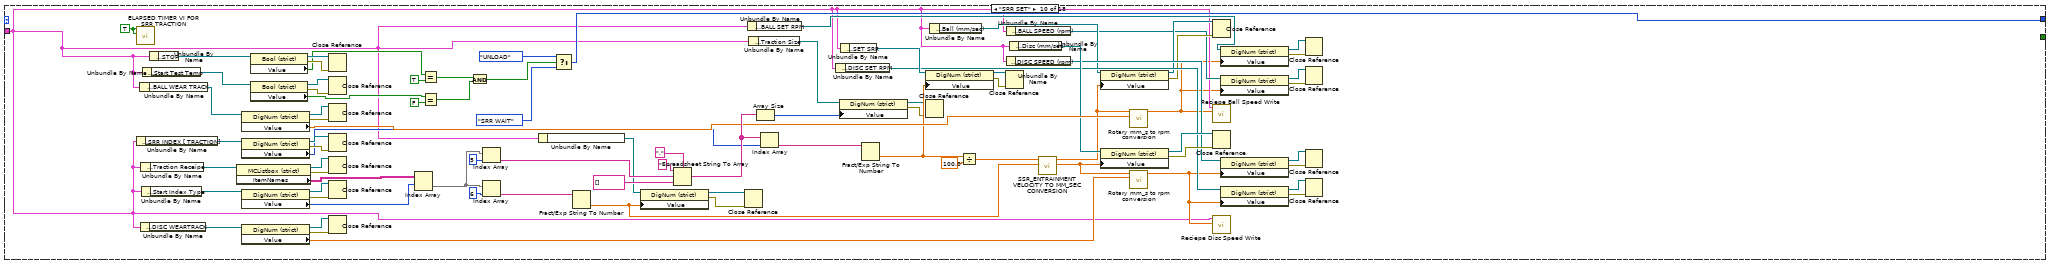
[diagram p12: hidden frame]
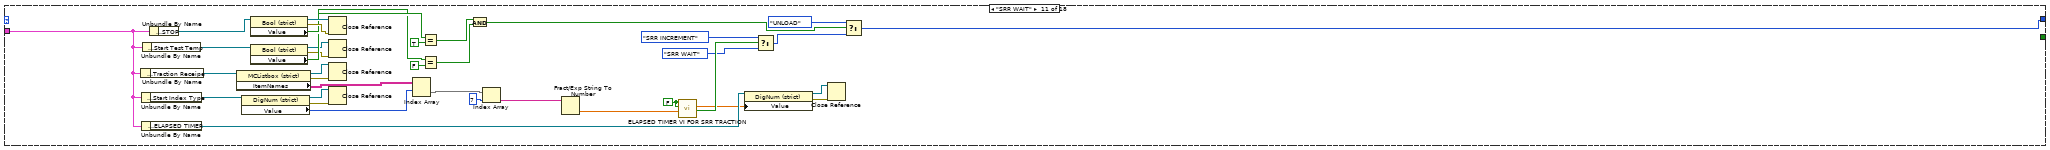
[diagram p13: hidden frame]
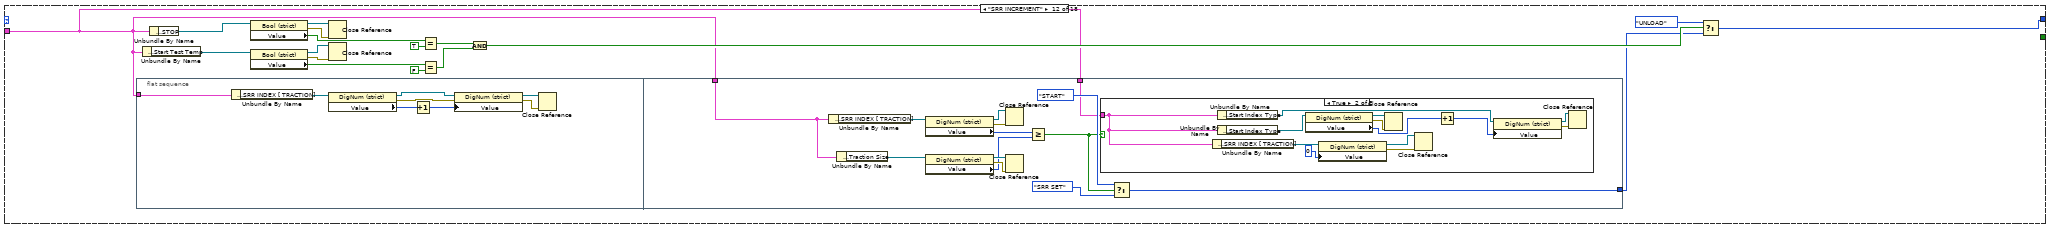
[diagram p14: hidden frame]
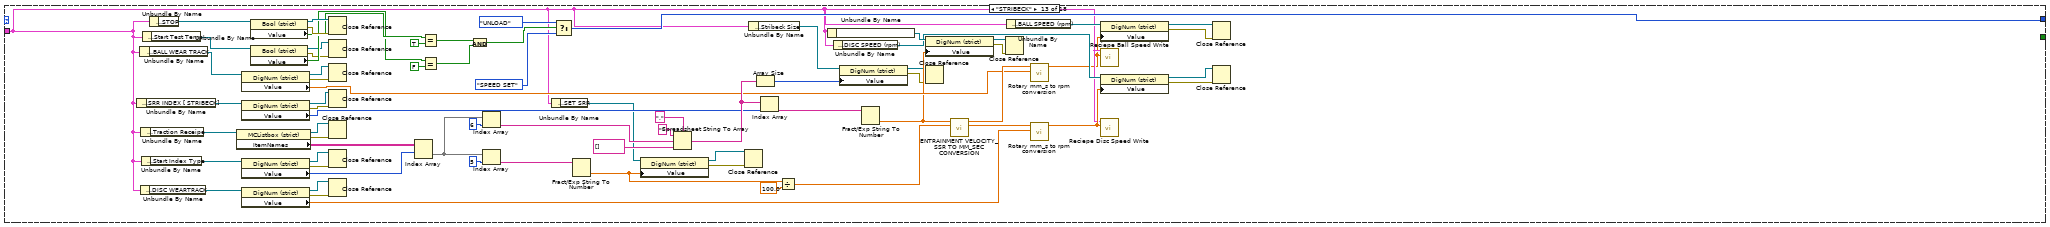
[diagram p16: hidden frame]
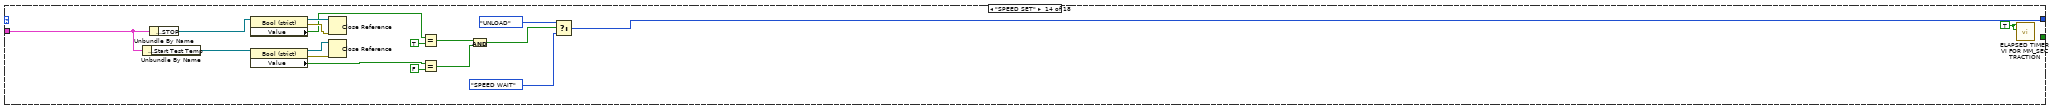
[diagram p17: hidden frame]
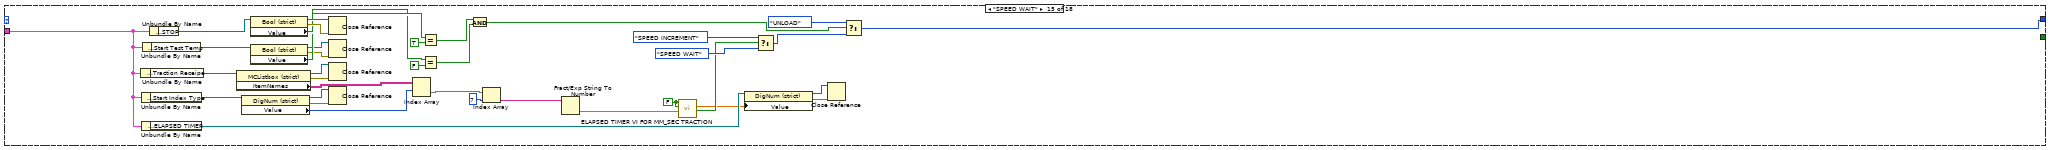
[diagram p18: hidden frame]
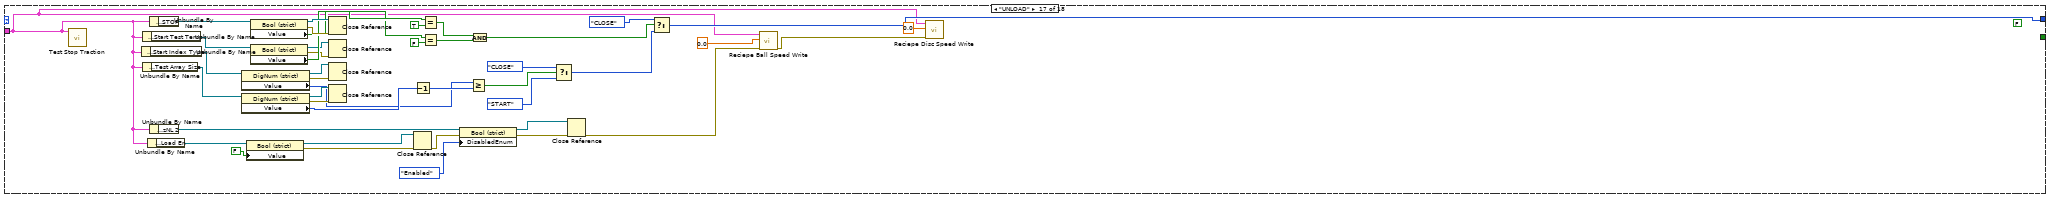
[diagram p20: hidden frame]
diagram:
  n1 = case shown="No Error" "error in (no error)" {
    tunnel: "main ref" -> [w4 _]
    frame No Error {
      n2 = Unbundle By Name(w4) -> ("Main Screen.Start Test Temp"=w15:refnum<vi>)
      n3 = Unbundle By Name(w4) -> ("Main Screen.Start Test"=w12:refnum<vi>)
      n4 = Unbundle By Name(w4) -> ("Motion Module.Traction"=w7:refnum<vi>)
      n5 = property class="Bool (strict)"(reference=w7) -> (reference out=w6:refnum<vi>, error out=w8:errorcluster, "Value"=w5:bool)  [unwired: 1 in]
      n6 = property class="Bool (strict)"(reference=w15) -> (reference out=w16:refnum<vi>, error out=w14:errorcluster, "Value"=w10:bool)  [unwired: 1 in]
      n7 = property class="Bool (strict)"(reference=w12) -> (reference out=w11:refnum<vi>, error out=w13:errorcluster, "Value"=w9:bool)  [unwired: 1 in]
      n8 = Close Reference(reference=w6, error in (no error)=w8) -> ()  [unwired: 1 out]
      n9 = Close Reference(reference=w16, error in (no error)=w14) -> ()  [unwired: 1 out]
      n10 = Close Reference(reference=w11, error in (no error)=w13) -> ()  [unwired: 1 out]
      n11 = Compound Arithmetic op=AND(w5, w10, w9) -> (w3:bool)
      n12 = case shown="True" w3 {
        tunnel: w4 -> [_ w17]
        frame False {
        }
        frame True {
          n13 = while {
            shift-right: [w26] -> _
            shift-left: "Enum - Menu" -> [w19]
            tunnel: w17 -> [w21]
            stop <- w25 stop-if-true
            n14 = Unbundle By Name(w21) -> ("Traction reciepe.Enum - Menu"=w22:refnum<vi>)
            n15 = case shown="\"SPEED INCREMENT\"" w19 {
              tunnel: [w64 w77 w147 w188 w206 w232 w251 w294 w324 w400 w440 w465 w559 w587 w618 w648 w738 Traction_Receipe_Enum."INIT" ("Enum - Menu")] -> w26
              tunnel: [w42 _ _ _ _ _ _ _ _ _ _ _ _ _ _ _ _ TRUE] -> w25
              tunnel: w21 -> [w28 w68 w106 w175 w208 w224 w253 w269 w314 w344 w428 w464 w517 w589 w606 w642 w718 w758]
              frame "INIT", Default {
                w27 = 0 ("Value")
                n16 = Unbundle By Name(w28) -> ("Traction reciepe.SRR INDEX [ TRACTION]"=w33:refnum<vi>)
                n17 = Unbundle By Name(w28) -> ("Traction reciepe.SRR INDEX [ STRIBECK]"=w36:refnum<vi>)
                n18 = Unbundle By Name(w28) -> ("Traction reciepe.Start Index Type"=w30:refnum<vi>)
                n19 = Unbundle By Name(w28) -> ("Main Screen.Start Test Temp"=w62:refnum<vi>)
                n20 = Unbundle By Name(w28) -> ("Main Screen.Start Test Temp"=w49:refnum<vi>)
                n21 = Unbundle By Name(w28) -> ("Main Screen.Start Test"=w59:refnum<vi>)
                n22 = Unbundle By Name(w28) -> ("Motion Module.Traction"=w40:refnum<vi>)
                n23 = Unbundle By Name(w28) -> ("Main Screen.STOP"=w52:refnum<vi>)
                n24 = property class="DigNum (strict)"(reference=w36, "Value"=w27) -> (reference out=w35:refnum<vi>, error out=w37:errorcluster)  [unwired: 1 in]
                n25 = property class="DigNum (strict)"(reference=w30, "Value"=w27) -> (reference out=w29:refnum<vi>, error out=w31:errorcluster)  [unwired: 1 in]
                n26 = property class="DigNum (strict)"(reference=w33, "Value"=w27) -> (reference out=w34:refnum<vi>, error out=w32:errorcluster)  [unwired: 1 in]
                n27 = property class="Bool (strict)"(reference=w40) -> (reference out=w39:refnum<vi>, error out=w41:errorcluster, "Value"=w38:bool)  [unwired: 1 in]
                n28 = property class="Bool (strict)"(reference=w62) -> (reference out=w63:refnum<vi>, error out=w61:errorcluster, "Value"=w57:bool)  [unwired: 1 in]
                n29 = property class="Bool (strict)"(reference=w59) -> (reference out=w58:refnum<vi>, error out=w60:errorcluster, "Value"=w56:bool)  [unwired: 1 in]
                n30 = property class="Bool (strict)"(reference=w52) -> (reference out=w54:refnum<vi>, error out=w53:errorcluster, "Value"=w51:bool)  [unwired: 1 in]
                n31 = property class="Bool (strict)"(reference=w49) -> (reference out=w47:refnum<vi>, error out=w48:errorcluster, "Value"=w50:bool)  [unwired: 1 in]
                n32 = Close Reference(reference=w39, error in (no error)=w41) -> ()  [unwired: 1 out]
                n33 = Close Reference(reference=w35, error in (no error)=w37) -> ()  [unwired: 1 out]
                n34 = Close Reference(reference=w63, error in (no error)=w61) -> ()  [unwired: 1 out]
                n35 = Close Reference(reference=w29, error in (no error)=w31) -> ()  [unwired: 1 out]
                n36 = Close Reference(reference=w58, error in (no error)=w60) -> ()  [unwired: 1 out]
                n37 = Close Reference(reference=w54, error in (no error)=w53) -> ()  [unwired: 1 out]
                n38 = Close Reference(reference=w34, error in (no error)=w32) -> ()  [unwired: 1 out]
                n39 = Close Reference(reference=w47, error in (no error)=w48) -> ()  [unwired: 1 out]
                n40 = Compound Arithmetic op=AND(w38, w57, w56) -> (w55:bool)
                n41 = Equal?(x=w51, y=TRUE) -> (x = y?=w46:bool)
                n42 = Equal?(x=w50, y=FALSE) -> (x = y?=w45:bool)
                n43 = And(x=w46, y=w45) -> (x .and. y?=w42:bool)
                n44 = Select(t=Traction_Receipe_Enum."START" ("Enum - Menu"), s=w55, f=Traction_Receipe_Enum."INIT" ("Enum - Menu")) -> (s? t:f=w64:T2)
              }
              frame "START" {
                n45 = Unbundle By Name(w68) -> ("Traction reciepe.Traction Receipe"=w95:refnum<vi>)
                n46 = Unbundle By Name(w68) -> ("Traction reciepe.Start Index Type"=w70:refnum<vi>)
                n47 = Unbundle By Name(w68) -> ("Main Screen.Start Test Temp"=w86:refnum<vi>)
                n48 = Unbundle By Name(w68) -> ("Traction reciepe.Test Array Size"=w74:refnum<vi>)
                n49 = Unbundle By Name(w68) -> ("Main Screen.STOP"=w89:refnum<vi>)
                n50 = property class="MCListbox (strict)"(reference=w95) -> (reference out=w93:refnum<vi>, error out=w94:errorcluster, "ItemNames"=w92:string[][])  [unwired: 1 in]
                n51 = property class="DigNum (strict)"(reference=w70) -> (reference out=w69:refnum<vi>, error out=w71:errorcluster, "Value"=w67:i32)  [unwired: 1 in]
                n52 = property class="Bool (strict)"(reference=w89) -> (reference out=w91:refnum<vi>, error out=w90:errorcluster, "Value"=w88:bool)  [unwired: 1 in]
                n53 = property class="Bool (strict)"(reference=w86) -> (reference out=w84:refnum<vi>, error out=w85:errorcluster, "Value"=w87:bool)  [unwired: 1 in]
                n54 = Close Reference(reference=w91, error in (no error)=w90) -> ()  [unwired: 1 out]
                n55 = Close Reference(reference=w93, error in (no error)=w94) -> ()  [unwired: 1 out]
                n56 = Close Reference(reference=w84, error in (no error)=w85) -> ()  [unwired: 1 out]
                n57 = Close Reference(reference=w69, error in (no error)=w71) -> ()  [unwired: 1 out]
                n58 = Index Array(array=w92, index (row)=w67) -> (element=w101:string[])  [unwired: 1 in]
                n59 = Index Array(array=w92, index (col)=0 ("index (row)")) -> (element=w97:string[])  [unwired: 1 in]
                n60 = Equal?(x=w88, y=TRUE) -> (x = y?=w83:bool)
                n61 = Equal?(x=w87, y=FALSE) -> (x = y?=w82:bool)
                n62 = Array Size(array=w97) -> (size(s)=w72:i32)
                n63 = And(x=w83, y=w82) -> (x .and. y?=w79:bool)
                n64 = Index Array(array=w101, index=1) -> (element=w103:string)
                n65 = Equal?(x=w103, y="\"TRACTION\"") -> (x = y?=w98:bool)
                n66 = property class="DigNum (strict)"(reference=w74, "Value"=w72) -> (reference out=w73:refnum<vi>, error out=w75:errorcluster)  [unwired: 1 in]
                n67 = Close Reference(reference=w73, error in (no error)=w75) -> ()  [unwired: 1 out]
                n68 = Select(t=Traction_Receipe_Enum."TRACTION" ("Enum - Menu"), s=w98, f=Traction_Receipe_Enum."STRIBECK" ("Enum - Menu")) -> (s? t:f=w78:T2)
                n69 = Select(t=Traction_Receipe_Enum."UNLOAD", s=w79, f=w78) -> (s? t:f=w77:T2)
              }
              frame "TRACTION" {
                n70 = Unbundle By Name(w106) -> ("Traction reciepe.SRR INDEX [ TRACTION]"=w129:refnum<vi>)
                n71 = Unbundle By Name(w106) -> ("Traction reciepe.BALL WEAR TRACK"=w133:refnum<vi>)
                n72 = Unbundle By Name(w106) -> ("Traction reciepe.DISC WEARTRACK"=w137:refnum<vi>)
                n73 = Unbundle By Name(w106) -> ("Traction reciepe.Traction Receipe"=w145:refnum<vi>)
                n74 = Unbundle By Name(w106) -> ("Traction reciepe.Start Index Type"=w140:refnum<vi>)
                n75 = Unbundle By Name(w106) -> ("Main Screen.Start Test Temp"=w156:refnum<vi>)
                n76 = Unbundle By Name(w106) -> ("Main Screen.STOP"=w159:refnum<vi>)
                n77 = property class="MCListbox (strict)"(reference=w145) -> (reference out=w143:refnum<vi>, error out=w144:errorcluster, "ItemNames"=w142:string[][])  [unwired: 1 in]
                n78 = property class="DigNum (strict)"(reference=w129) -> (reference out=w127:refnum<vi>, error out=w128:errorcluster, "Value"=w126:i32)  [unwired: 1 in]
                n79 = property class="DigNum (strict)"(reference=w140) -> (reference out=w139:refnum<vi>, error out=w141:errorcluster, "Value"=w138:i32)  [unwired: 1 in]
                n80 = property class="DigNum (strict)"(reference=w133) -> (reference out=w131:refnum<vi>, error out=w132:errorcluster, "Value"=w130:dbl)  [unwired: 1 in]
                n81 = property class="DigNum (strict)"(reference=w137) -> (reference out=w135:refnum<vi>, error out=w136:errorcluster, "Value"=w134:dbl)  [unwired: 1 in]
                n82 = property class="Bool (strict)"(reference=w159) -> (reference out=w161:refnum<vi>, error out=w160:errorcluster, "Value"=w158:bool)  [unwired: 1 in]
                n83 = property class="Bool (strict)"(reference=w156) -> (reference out=w154:refnum<vi>, error out=w155:errorcluster, "Value"=w157:bool)  [unwired: 1 in]
                n84 = Close Reference(reference=w161, error in (no error)=w160) -> ()  [unwired: 1 out]
                n85 = Close Reference(reference=w154, error in (no error)=w155) -> ()  [unwired: 1 out]
                n86 = Close Reference(reference=w127, error in (no error)=w128) -> ()  [unwired: 1 out]
                n87 = Close Reference(reference=w143, error in (no error)=w144) -> ()  [unwired: 1 out]
                n88 = Close Reference(reference=w139, error in (no error)=w141) -> ()  [unwired: 1 out]
                n89 = Close Reference(reference=w131, error in (no error)=w132) -> ()  [unwired: 1 out]
                n90 = Close Reference(reference=w135, error in (no error)=w136) -> ()  [unwired: 1 out]
                n91 = Index Array(array=w142, index (row)=w138) -> (element=w168:string[])  [unwired: 1 in]
                n92 = Equal?(x=w158, y=TRUE) -> (x = y?=w153:bool)
                n93 = Equal?(x=w157, y=FALSE) -> (x = y?=w152:bool)
                n94 = And(x=w153, y=w152) -> (x .and. y?=w149:bool)
                n95 = Index Array(array=w168, index=5) -> (element=w167:string)
                n96 = Index Array(array=w168, index=6) -> (element=w163:string)
                n97 = Select(t=Traction_Receipe_Enum."UNLOAD", s=w149, f=Traction_Receipe_Enum."TEMPERATURE SET" ("Enum - Menu")) -> (s? t:f=w147:T2)
                n98 = Fract/Exp String To Number(string=w163) -> (number=w166:dbl)  [unwired: 3 in, 1 out]
                n99 = Unbundle By Name(w106) -> ("Traction reciepe.Ball (mm/sec)"=w111:refnum<vi>)
                n100 = Spreadsheet String To Array(delimiter (Tab)=",", format string="", spreadsheet string=w167, array type (2D Dbl)=string[] []) -> (array=w162:string[])
                n101 = Unbundle By Name(w106) -> ("Traction reciepe.BALL SPEED (rpm)"=w118:refnum<vi>)
                n102 = Unbundle By Name(w106) -> ("Traction reciepe.Traction Size"=w125:refnum<vi>)
                n103 = Array Size(array=w162) -> (size(s)=w122:i32)
                n104 = Index Array(array=w162, index=w126) -> (element=w164:string)
                n105 = Unbundle By Name(w106) -> ("Traction reciepe.Ball (mm/sec)"=w107:refnum<vi>)
                n106 = property class="DigNum (strict)"(reference=w125, "Value"=w122) -> (reference out=w123:refnum<vi>, error out=w124:errorcluster)  [unwired: 1 in]
                n107 = Fract/Exp String To Number(string=w164) -> (number=w165:dbl)  [unwired: 3 in, 1 out]
                n108 = Close Reference(reference=w123, error in (no error)=w124) -> ()  [unwired: 1 out]
                n109 = Unbundle By Name(w106) -> ("Traction reciepe.DISC SPEED (rpm)"=w119:refnum<vi>)
                n110 = call "SSR_ENTRAINMENT VELOCITY TO MM_SEC CONVERSION.vi"("Entrainment Speed"=w166, "Initial SSR"=w165) -> ("Disc"=w105:dbl, "Ball"=w110:dbl)  [unwired: 7 in, 1 out]
                n111 = property class="DigNum (strict)"(reference=w111, "Value"=w110) -> (reference out=w113:refnum<vi>, error out=w112:errorcluster)  [unwired: 1 in]
                n112 = property class="DigNum (strict)"(reference=w107, "Value"=w105) -> (reference out=w109:refnum<vi>, error out=w108:errorcluster)  [unwired: 1 in]
                n113 = call "Rotary mm_s to rpm conversion.vi"("Wear Track Diameter"=w130, "Enter initial Velocity (m/s)  3"=w110) -> ("Initial Speed (RPM) 2"=w115:dbl)  [unwired: 7 in, 2 out]
                n114 = call "Rotary mm_s to rpm conversion.vi"("Wear Track Diameter"=w134, "Enter initial Velocity (m/s)  3"=w105) -> ("Initial Speed (RPM) 2"=w114:dbl)  [unwired: 7 in, 2 out]
                n115 = Close Reference(reference=w113, error in (no error)=w112) -> ()  [unwired: 1 out]
                n116 = Close Reference(reference=w109, error in (no error)=w108) -> ()  [unwired: 1 out]
                n117 = property class="DigNum (strict)"(reference=w118, "Value"=w115) -> (reference out=w116:refnum<vi>, error out=w117:errorcluster)  [unwired: 1 in]
                n118 = property class="DigNum (strict)"(reference=w119, "Value"=w114) -> (reference out=w121:refnum<vi>, error out=w120:errorcluster)  [unwired: 1 in]
                n119 = Close Reference(reference=w116, error in (no error)=w117) -> ()  [unwired: 1 out]
                n120 = Close Reference(reference=w121, error in (no error)=w120) -> ()  [unwired: 1 out]
              }
              frame "TEMPERATURE SET" {
                n121 = Unbundle By Name(w175) -> ("Traction reciepe.Traction Receipe"=w186:refnum<vi>)
                n122 = Unbundle By Name(w175) -> ("Traction reciepe.Start Index Type"=w181:refnum<vi>)
                n123 = Unbundle By Name(w175) -> ("Main Screen.Start Test Temp"=w197:refnum<vi>)
                n124 = Unbundle By Name(w175) -> ("Main Screen.STOP"=w200:refnum<vi>)
                n125 = property class="MCListbox (strict)"(reference=w186) -> (reference out=w184:refnum<vi>, error out=w185:errorcluster, "ItemNames"=w183:string[][])  [unwired: 1 in]
                n126 = property class="DigNum (strict)"(reference=w181) -> (reference out=w180:refnum<vi>, error out=w182:errorcluster, "Value"=w179:i32)  [unwired: 1 in]
                n127 = property class="Bool (strict)"(reference=w200) -> (reference out=w202:refnum<vi>, error out=w201:errorcluster, "Value"=w199:bool)  [unwired: 1 in]
                n128 = property class="Bool (strict)"(reference=w197) -> (reference out=w195:refnum<vi>, error out=w196:errorcluster, "Value"=w198:bool)  [unwired: 1 in]
                n129 = Close Reference(reference=w184, error in (no error)=w185) -> ()  [unwired: 1 out]
                n130 = Close Reference(reference=w180, error in (no error)=w182) -> ()  [unwired: 1 out]
                n131 = Close Reference(reference=w202, error in (no error)=w201) -> ()  [unwired: 1 out]
                n132 = Close Reference(reference=w195, error in (no error)=w196) -> ()  [unwired: 1 out]
                n133 = Index Array(array=w183, index (row)=w179) -> (element=w205:string[])  [unwired: 1 in]
                n134 = Equal?(x=w199, y=TRUE) -> (x = y?=w194:bool)
                n135 = Equal?(x=w198, y=FALSE) -> (x = y?=w193:bool)
                n136 = And(x=w194, y=w193) -> (x .and. y?=w190:bool)
                n137 = Index Array(array=w205, index=3) -> (element=w203:string)
                n138 = Unbundle By Name(w175) -> ("Traction reciepe.SET TEMPERATURE"=w177:refnum<vi>)
                n139 = Select(t=Traction_Receipe_Enum."UNLOAD", s=w190, f=Traction_Receipe_Enum."CHURNING START" ("Enum - Menu")) -> (s? t:f=w188:T2)
                n140 = Fract/Exp String To Number(string=w203) -> (number=w174:dbl)  [unwired: 3 in, 1 out]
                n141 = property class="DigNum (strict)"(reference=w177, "Value"=w174) -> (reference out=w176:refnum<vi>, error out=w178:errorcluster)  [unwired: 1 in]
                n142 = Close Reference(reference=w176, error in (no error)=w178) -> ()  [unwired: 1 out]
              }
              frame "CHURNING START" {
                n143 = Unbundle By Name(w208) -> ("Main Screen.Start Test Temp"=w217:refnum<vi>)
                n144 = Unbundle By Name(w208) -> ("Main Screen.STOP"=w220:refnum<vi>)
                n145 = property class="Bool (strict)"(reference=w220) -> (reference out=w222:refnum<vi>, error out=w221:errorcluster, "Value"=w219:bool)  [unwired: 1 in]
                n146 = property class="Bool (strict)"(reference=w217) -> (reference out=w215:refnum<vi>, error out=w216:errorcluster, "Value"=w218:bool)  [unwired: 1 in]
                n147 = Close Reference(reference=w222, error in (no error)=w221) -> ()  [unwired: 1 out]
                n148 = Close Reference(reference=w215, error in (no error)=w216) -> ()  [unwired: 1 out]
                n149 = Equal?(x=w219, y=TRUE) -> (x = y?=w214:bool)
                n150 = Equal?(x=w218, y=FALSE) -> (x = y?=w213:bool)
                n151 = And(x=w214, y=w213) -> (x .and. y?=w210:bool)
                n152 = Select(t=Traction_Receipe_Enum."UNLOAD", s=w210, f=Traction_Receipe_Enum."TEMPERATURE REACH" ("Enum - Menu")) -> (s? t:f=w206:T2)
              }
              frame "TEMPERATURE REACH" {
                n153 = Unbundle By Name(w224) -> ("Traction reciepe.TEMPERATURE READ"=w231:refnum<vi>)
                n154 = Unbundle By Name(w224) -> ("Traction reciepe.SET TEMPERATURE"=w225:refnum<vi>)
                n155 = Unbundle By Name(w224) -> ("Main Screen.Start Test Temp"=w242:refnum<vi>)
                n156 = Unbundle By Name(w224) -> ("Main Screen.STOP"=w245:refnum<vi>)
                n157 = property class="DigNum (strict)"(reference=w231) -> (reference out=w229:refnum<vi>, error out=w230:errorcluster, "Value"=w228:dbl)  [unwired: 1 in]
                n158 = property class="DigNum (strict)"(reference=w225) -> (reference out=w227:refnum<vi>, error out=w226:errorcluster, "Value"=w223:dbl)  [unwired: 1 in]
                n159 = property class="Bool (strict)"(reference=w245) -> (reference out=w247:refnum<vi>, error out=w246:errorcluster, "Value"=w244:bool)  [unwired: 1 in]
                n160 = property class="Bool (strict)"(reference=w242) -> (reference out=w240:refnum<vi>, error out=w241:errorcluster, "Value"=w243:bool)  [unwired: 1 in]
                n161 = Close Reference(reference=w247, error in (no error)=w246) -> ()  [unwired: 1 out]
                n162 = Close Reference(reference=w240, error in (no error)=w241) -> ()  [unwired: 1 out]
                n163 = Close Reference(reference=w229, error in (no error)=w230) -> ()  [unwired: 1 out]
                n164 = Close Reference(reference=w227, error in (no error)=w226) -> ()  [unwired: 1 out]
                n165 = Greater Or Equal?(x=w228, y=w223) -> (x >= y?=w250:bool)
                n166 = Equal?(x=w244, y=TRUE) -> (x = y?=w239:bool)
                n167 = Equal?(x=w243, y=FALSE) -> (x = y?=w238:bool)
                n168 = Select(t=Traction_Receipe_Enum."CHURNING STOP" ("Enum - Menu"), s=w250, f=Traction_Receipe_Enum."TEMPERATURE REACH" ("Enum - Menu")) -> (s? t:f=w233:T2)
                n169 = And(x=w239, y=w238) -> (x .and. y?=w235:bool)
                n170 = Select(t=Traction_Receipe_Enum."UNLOAD", s=w235, f=w233) -> (s? t:f=w232:T2)
              }
              frame "CHURNING STOP" {
                n171 = Unbundle By Name(w253) -> ("Main Screen.Start Test Temp"=w262:refnum<vi>)
                n172 = Unbundle By Name(w253) -> ("Main Screen.STOP"=w265:refnum<vi>)
                n173 = property class="Bool (strict)"(reference=w265) -> (reference out=w267:refnum<vi>, error out=w266:errorcluster, "Value"=w264:bool)  [unwired: 1 in]
                n174 = property class="Bool (strict)"(reference=w262) -> (reference out=w260:refnum<vi>, error out=w261:errorcluster, "Value"=w263:bool)  [unwired: 1 in]
                n175 = Close Reference(reference=w267, error in (no error)=w266) -> ()  [unwired: 1 out]
                n176 = Close Reference(reference=w260, error in (no error)=w261) -> ()  [unwired: 1 out]
                n177 = Equal?(x=w264, y=TRUE) -> (x = y?=w259:bool)
                n178 = Equal?(x=w263, y=FALSE) -> (x = y?=w258:bool)
                n179 = And(x=w259, y=w258) -> (x .and. y?=w255:bool)
                n180 = Select(t=Traction_Receipe_Enum."UNLOAD", s=w255, f=Traction_Receipe_Enum."LOAD" ("Enum - Menu")) -> (s? t:f=w251:T2)
              }
              frame "LOAD" {
                n181 = Unbundle By Name(w269) -> ("Traction reciepe.Traction Receipe"=w293:refnum<vi>)
                n182 = Unbundle By Name(w269) -> ("Traction reciepe.Start Index Type"=w275:refnum<vi>)
                n183 = Unbundle By Name(w269) -> ("Main Screen.Start Test Temp"=w304:refnum<vi>)
                n184 = Unbundle By Name(w269) -> ("Main Screen.STOP"=w307:refnum<vi>)
                n185 = property class="MCListbox (strict)"(reference=w293) -> (reference out=w291:refnum<vi>, error out=w292:errorcluster, "ItemNames"=w290:string[][])  [unwired: 1 in]
                n186 = property class="DigNum (strict)"(reference=w275) -> (reference out=w274:refnum<vi>, error out=w276:errorcluster, "Value"=w273:i32)  [unwired: 1 in]
                n187 = property class="Bool (strict)"(reference=w307) -> (reference out=w309:refnum<vi>, error out=w308:errorcluster, "Value"=w306:bool)  [unwired: 1 in]
                n188 = property class="Bool (strict)"(reference=w304) -> (reference out=w302:refnum<vi>, error out=w303:errorcluster, "Value"=w305:bool)  [unwired: 1 in]
                n189 = Close Reference(reference=w309, error in (no error)=w308) -> ()  [unwired: 1 out]
                n190 = Close Reference(reference=w302, error in (no error)=w303) -> ()  [unwired: 1 out]
                n191 = Close Reference(reference=w291, error in (no error)=w292) -> ()  [unwired: 1 out]
                n192 = Close Reference(reference=w274, error in (no error)=w276) -> ()  [unwired: 1 out]
                n193 = Index Array(array=w290, index (row)=w273) -> (element=w312:string[])  [unwired: 1 in]
                n194 = Equal?(x=w306, y=TRUE) -> (x = y?=w301:bool)
                n195 = Equal?(x=w305, y=FALSE) -> (x = y?=w300:bool)
                n196 = And(x=w301, y=w300) -> (x .and. y?=w297:bool)
                n197 = Index Array(array=w312, index=4) -> (element=w311:string)
                n198 = Unbundle By Name(w269) -> ("Main Screen.Set Load (N)"=w279:refnum<vi>)
                n199 = Unbundle By Name(w269) -> ("Traction reciepe.SET LOAD"=w271:refnum<vi>)
                n200 = Select(t=Traction_Receipe_Enum."UNLOAD", s=w297, f=Traction_Receipe_Enum."LOAD REACHED" ("Enum - Menu")) -> (s? t:f=w294:T2)
                n201 = Fract/Exp String To Number(string=w311) -> (number=w268:dbl)  [unwired: 3 in, 1 out]
                n202 = property class="DigNum (strict)"(reference=w279, "Value"=w268) -> (reference out=w278:refnum<vi>, error out=w280:errorcluster)  [unwired: 1 in]
                n203 = property class="DigNum (strict)"(reference=w271, "Value"=w268) -> (reference out=w270:refnum<vi>, error out=w272:errorcluster)  [unwired: 1 in]
                n204 = Unbundle By Name(w269) -> ("Main Screen.Load En"=w289:refnum<vi>)
                n205 = Close Reference(reference=w270, error in (no error)=w272) -> ()  [unwired: 1 out]
                n206 = Close Reference(reference=w278, error in (no error)=w280) -> (error out=w277:errorcluster)
                n207 = property on="Property Node" class="Bool (strict)"(reference=w289, error in=w277, "Value"=TRUE) -> (reference out=w287:refnum<vi>, error out=w288:errorcluster)
                n208 = Unbundle By Name(w269) -> ("Main Screen.zNL 2"=w284:refnum<vi>)
                n209 = Close Reference(reference=w287, error in (no error)=w288) -> (error out=w283:errorcluster)
                n210 = property on="Property Node" class="Bool (strict)"(reference=w284, error in=w283, "DisabledEnum"=T3."Disabled and Grayed Out" ("Disabled")) -> (reference out=w286:refnum<vi>, error out=w285:errorcluster)
                n211 = Close Reference(reference=w286, error in (no error)=w285) -> ()  [unwired: 1 out]
              }
              frame "LOAD REACHED" {
                n212 = Unbundle By Name(w314) -> ("Main Screen.Start Test Temp"=w334:refnum<vi>)
                n213 = Unbundle By Name(w314) -> ("Main Screen.NL Display 4"=w321:refnum<vi>)
                n214 = Unbundle By Name(w314) -> ("Traction reciepe.SET LOAD"=w315:refnum<vi>)
                n215 = Unbundle By Name(w314) -> ("Main Screen.STOP"=w337:refnum<vi>)
                n216 = property class="DigNum (strict)"(reference=w321) -> (reference out=w323:refnum<vi>, error out=w322:errorcluster, "Value"=w320:dbl)  [unwired: 1 in]
                n217 = property class="DigNum (strict)"(reference=w315) -> (reference out=w317:refnum<vi>, error out=w316:errorcluster, "Value"=w313:dbl)  [unwired: 1 in]
                n218 = property class="Bool (strict)"(reference=w337) -> (reference out=w339:refnum<vi>, error out=w338:errorcluster, "Value"=w336:bool)  [unwired: 1 in]
                n219 = property class="Bool (strict)"(reference=w334) -> (reference out=w332:refnum<vi>, error out=w333:errorcluster, "Value"=w335:bool)  [unwired: 1 in]
                n220 = Close Reference(reference=w339, error in (no error)=w338) -> ()  [unwired: 1 out]
                n221 = Close Reference(reference=w332, error in (no error)=w333) -> ()  [unwired: 1 out]
                n222 = Close Reference(reference=w323, error in (no error)=w322) -> ()  [unwired: 1 out]
                n223 = Close Reference(reference=w317, error in (no error)=w316) -> ()  [unwired: 1 out]
                n224 = Equal?(x=w336, y=TRUE) -> (x = y?=w331:bool)
                n225 = Equal?(x=w335, y=FALSE) -> (x = y?=w330:bool)
                n226 = Subtract(x=w313, y=0.4) -> (x-y=w319:dbl)
                n227 = Greater Or Equal?(x=w320, y=w319) -> (x >= y?=w342:bool)
                n228 = And(x=w331, y=w330) -> (x .and. y?=w327:bool)
                n229 = Select(t=Traction_Receipe_Enum."SRR SET" ("Enum - Menu"), s=w342, f=Traction_Receipe_Enum."LOAD REACHED" ("Enum - Menu")) -> (s? t:f=w325:T2)
                n230 = Select(t=Traction_Receipe_Enum."UNLOAD", s=w327, f=w325) -> (s? t:f=w324:T2)
              }
              frame "SRR SET" {
                w426 = TRUE ("PAUSE")
                n231 = call "ELAPSED TIMER VI FOR SRR TRACTION.vi"("RESET"=w426, "PAUSE"=w426) -> ()  [unwired: 7 in, 3 out]
                n232 = Unbundle By Name(w344) -> ("Traction reciepe.SRR INDEX [ TRACTION]"=w369:refnum<vi>)
                n233 = Unbundle By Name(w344) -> ("Traction reciepe.BALL WEAR TRACK"=w385:refnum<vi>)
                n234 = Unbundle By Name(w344) -> ("Traction reciepe.DISC WEARTRACK"=w389:refnum<vi>)
                n235 = Unbundle By Name(w344) -> ("Traction reciepe.Traction Receipe"=w399:refnum<vi>)
                n236 = Unbundle By Name(w344) -> ("Traction reciepe.Start Index Type"=w392:refnum<vi>)
                n237 = Unbundle By Name(w344) -> ("Main Screen.Start Test Temp"=w410:refnum<vi>)
                n238 = Unbundle By Name(w344) -> ("Main Screen.STOP"=w413:refnum<vi>)
                n239 = property class="MCListbox (strict)"(reference=w399) -> (reference out=w397:refnum<vi>, error out=w398:errorcluster, "ItemNames"=w396:string[][])  [unwired: 1 in]
                n240 = property class="DigNum (strict)"(reference=w385) -> (reference out=w383:refnum<vi>, error out=w384:errorcluster, "Value"=w382:dbl)  [unwired: 1 in]
                n241 = property class="DigNum (strict)"(reference=w369) -> (reference out=w367:refnum<vi>, error out=w368:errorcluster, "Value"=w366:i32)  [unwired: 1 in]
                n242 = property class="DigNum (strict)"(reference=w392) -> (reference out=w391:refnum<vi>, error out=w393:errorcluster, "Value"=w390:i32)  [unwired: 1 in]
                n243 = property class="DigNum (strict)"(reference=w389) -> (reference out=w387:refnum<vi>, error out=w388:errorcluster, "Value"=w386:dbl)  [unwired: 1 in]
                n244 = property class="Bool (strict)"(reference=w413) -> (reference out=w415:refnum<vi>, error out=w414:errorcluster, "Value"=w412:bool)  [unwired: 1 in]
                n245 = property class="Bool (strict)"(reference=w410) -> (reference out=w408:refnum<vi>, error out=w409:errorcluster, "Value"=w411:bool)  [unwired: 1 in]
                n246 = Close Reference(reference=w415, error in (no error)=w414) -> ()  [unwired: 1 out]
                n247 = Close Reference(reference=w408, error in (no error)=w409) -> ()  [unwired: 1 out]
                n248 = Close Reference(reference=w383, error in (no error)=w384) -> ()  [unwired: 1 out]
                n249 = Close Reference(reference=w367, error in (no error)=w368) -> ()  [unwired: 1 out]
                n250 = Close Reference(reference=w397, error in (no error)=w398) -> ()  [unwired: 1 out]
                n251 = Close Reference(reference=w391, error in (no error)=w393) -> ()  [unwired: 1 out]
                n252 = Close Reference(reference=w387, error in (no error)=w388) -> ()  [unwired: 1 out]
                n253 = Index Array(array=w396, index (row)=w390) -> (element=w425:string[])  [unwired: 1 in]
                n254 = Equal?(x=w412, y=TRUE) -> (x = y?=w407:bool)
                n255 = Equal?(x=w411, y=FALSE) -> (x = y?=w406:bool)
                n256 = And(x=w407, y=w406) -> (x .and. y?=w403:bool)
                n257 = Index Array(array=w425, index=5) -> (element=w424:string)
                n258 = Index Array(array=w425, index=6) -> (element=w422:string)
                n259 = Unbundle By Name(w344) -> ("Traction reciepe.SET entrainment Velocity"=w377:refnum<vi>)
                n260 = Select(t=Traction_Receipe_Enum."UNLOAD", s=w403, f=Traction_Receipe_Enum."SRR WAIT" ("Enum - Menu")) -> (s? t:f=w400:T2)
                n261 = Fract/Exp String To Number(string=w422) -> (number=w374:dbl)  [unwired: 3 in, 1 out]
                n262 = property class="DigNum (strict)"(reference=w377, "Value"=w374) -> (reference out=w375:refnum<vi>, error out=w376:errorcluster)  [unwired: 1 in]
                n263 = Spreadsheet String To Array(delimiter (Tab)=",", format string="", spreadsheet string=w424, array type (2D Dbl)=string[] []) -> (array=w421:string[])
                n264 = Close Reference(reference=w375, error in (no error)=w376) -> ()  [unwired: 1 out]
                n265 = Unbundle By Name(w344) -> ("Traction reciepe.BALL SET RPM"=w354:refnum<vi>)
                n266 = Unbundle By Name(w344) -> ("Traction reciepe.Traction Size"=w373:refnum<vi>)
                n267 = Array Size(array=w421) -> (size(s)=w370:i32)
                n268 = Index Array(array=w421, index=w366) -> (element=w423:string)
                n269 = Unbundle By Name(w344) -> ("Traction reciepe.DISC SET RPM"=w358:refnum<vi>)
                n270 = property class="DigNum (strict)"(reference=w373, "Value"=w370) -> (reference out=w371:refnum<vi>, error out=w372:errorcluster)  [unwired: 1 in]
                n271 = Unbundle By Name(w344) -> ("Traction reciepe.SET SRR"=w381:refnum<vi>)
                n272 = Fract/Exp String To Number(string=w423) -> (number=w378:dbl)  [unwired: 3 in, 1 out]
                n273 = property class="DigNum (strict)"(reference=w381, "Value"=w378) -> (reference out=w379:refnum<vi>, error out=w380:errorcluster)  [unwired: 1 in]
                n274 = Close Reference(reference=w371, error in (no error)=w372) -> ()  [unwired: 1 out]
                n275 = Unbundle By Name(w344) -> ("Traction reciepe.Ball (mm/sec)"=w349:refnum<vi>)
                n276 = Divide(x=w378, y=100.0) -> (x/y=w395:dbl)
                n277 = Close Reference(reference=w379, error in (no error)=w380) -> ()  [unwired: 1 out]
                n278 = Unbundle By Name(w344) -> ("Traction reciepe.BALL SPEED (rpm)"=w347:refnum<vi>)
                n279 = Unbundle By Name(w344) -> ("Traction reciepe.DISC SPEED (rpm)"=w359:refnum<vi>)
                n280 = Unbundle By Name(w344) -> ("Traction reciepe.Disc (mm/sec)"=w365:refnum<vi>)
                n281 = call "SSR_ENTRAINMENT VELOCITY TO MM_SEC CONVERSION.vi"("Entrainment Speed"=w374, "Initial SSR"=w395) -> ("Disc"=w362:dbl, "Ball"=w348:dbl)  [unwired: 7 in, 1 out]
                n282 = property class="DigNum (strict)"(reference=w349, "Value"=w348) -> (reference out=w351:refnum<vi>, error out=w350:errorcluster)  [unwired: 1 in]
                n283 = property class="DigNum (strict)"(reference=w365, "Value"=w362) -> (reference out=w363:refnum<vi>, error out=w364:errorcluster)  [unwired: 1 in]
                n284 = call "Rotary mm_s to rpm conversion.vi"("Wear Track Diameter"=w382, "Enter initial Velocity (m/s)  3"=w348) -> ("Initial Speed (RPM) 2"=w343:dbl)  [unwired: 7 in, 2 out]
                n285 = call "Rotary mm_s to rpm conversion.vi"("Wear Track Diameter"=w386, "Enter initial Velocity (m/s)  3"=w362) -> ("Initial Speed (RPM) 2"=w355:dbl)  [unwired: 7 in, 2 out]
                n286 = Close Reference(reference=w351, error in (no error)=w350) -> ()  [unwired: 1 out]
                n287 = call "Reciepe Ball Speed Write.vi"("Set Speed"=w343, "main ref"=w344) -> ()  [unwired: 9 in, 1 out]
                n288 = Close Reference(reference=w363, error in (no error)=w364) -> ()  [unwired: 1 out]
                n289 = call "Reciepe Disc Speed Write.vi"("Set Speed"=w355, "main ref"=w344) -> ()  [unwired: 9 in, 1 out]
                n290 = property class="DigNum (strict)"(reference=w354, "Value"=w343) -> (reference out=w352:refnum<vi>, error out=w353:errorcluster)  [unwired: 1 in]
                n291 = property class="DigNum (strict)"(reference=w347, "Value"=w343) -> (reference out=w345:refnum<vi>, error out=w346:errorcluster)  [unwired: 1 in]
                n292 = property class="DigNum (strict)"(reference=w359, "Value"=w355) -> (reference out=w361:refnum<vi>, error out=w360:errorcluster)  [unwired: 1 in]
                n293 = property class="DigNum (strict)"(reference=w358, "Value"=w355) -> (reference out=w356:refnum<vi>, error out=w357:errorcluster)  [unwired: 1 in]
                n294 = Close Reference(reference=w352, error in (no error)=w353) -> ()  [unwired: 1 out]
                n295 = Close Reference(reference=w345, error in (no error)=w346) -> ()  [unwired: 1 out]
                n296 = Close Reference(reference=w361, error in (no error)=w360) -> ()  [unwired: 1 out]
                n297 = Close Reference(reference=w356, error in (no error)=w357) -> ()  [unwired: 1 out]
              }
              frame "SRR WAIT" {
                w460 = FALSE ("PAUSE")
                n298 = Unbundle By Name(w428) -> ("Traction reciepe.Traction Receipe"=w439:refnum<vi>)
                n299 = Unbundle By Name(w428) -> ("Traction reciepe.Start Index Type"=w434:refnum<vi>)
                n300 = Unbundle By Name(w428) -> ("Traction reciepe.ELAPSED TIMER"=w431:refnum<vi>)
                n301 = Unbundle By Name(w428) -> ("Main Screen.Start Test Temp"=w450:refnum<vi>)
                n302 = Unbundle By Name(w428) -> ("Main Screen.STOP"=w453:refnum<vi>)
                n303 = property class="MCListbox (strict)"(reference=w439) -> (reference out=w437:refnum<vi>, error out=w438:errorcluster, "ItemNames"=w436:string[][])  [unwired: 1 in]
                n304 = property class="DigNum (strict)"(reference=w434) -> (reference out=w433:refnum<vi>, error out=w435:errorcluster, "Value"=w432:i32)  [unwired: 1 in]
                n305 = property class="Bool (strict)"(reference=w453) -> (reference out=w455:refnum<vi>, error out=w454:errorcluster, "Value"=w452:bool)  [unwired: 1 in]
                n306 = property class="Bool (strict)"(reference=w450) -> (reference out=w448:refnum<vi>, error out=w449:errorcluster, "Value"=w451:bool)  [unwired: 1 in]
                n307 = Close Reference(reference=w455, error in (no error)=w454) -> ()  [unwired: 1 out]
                n308 = Close Reference(reference=w448, error in (no error)=w449) -> ()  [unwired: 1 out]
                n309 = Close Reference(reference=w437, error in (no error)=w438) -> ()  [unwired: 1 out]
                n310 = Close Reference(reference=w433, error in (no error)=w435) -> ()  [unwired: 1 out]
                n311 = Index Array(array=w436, index (row)=w432) -> (element=w463:string[])  [unwired: 1 in]
                n312 = Equal?(x=w452, y=TRUE) -> (x = y?=w447:bool)
                n313 = Equal?(x=w451, y=FALSE) -> (x = y?=w446:bool)
                n314 = And(x=w447, y=w446) -> (x .and. y?=w443:bool)
                n315 = Index Array(array=w463, index=7) -> (element=w462:string)
                n316 = Fract/Exp String To Number(string=w462) -> (number=w459:dbl)  [unwired: 3 in, 1 out]
                n317 = call "ELAPSED TIMER VI FOR SRR TRACTION.vi"("TARGET"=w459, "RESET"=w460, "PAUSE"=w460) -> ("ELAPSED INDICATION"=w458:bool, "ELAPSED TIMER"=w427:dbl)  [unwired: 6 in, 1 out]
                n318 = property class="DigNum (strict)"(reference=w431, "Value"=w427) -> (reference out=w429:refnum<vi>, error out=w430:errorcluster)  [unwired: 1 in]
                n319 = Select(t=Traction_Receipe_Enum."SRR INCREMENT" ("Enum - Menu"), s=w458, f=Traction_Receipe_Enum."SRR WAIT") -> (s? t:f=w441:T2)
                n320 = Close Reference(reference=w429, error in (no error)=w430) -> ()  [unwired: 1 out]
                n321 = Select(t=Traction_Receipe_Enum."UNLOAD", s=w443, f=w441) -> (s? t:f=w440:T2)
              }
              frame "SRR INCREMENT" {
                n322 = flat-sequence {
                  tunnel: w464 -> [w487]
                  tunnel: [w500] -> w466
                  tunnel: w464 -> [w498]
                  tunnel: w464 -> [w490]
                  frame #0 {
                    n323 = Unbundle By Name(w487) -> ("Traction reciepe.SRR INDEX [ TRACTION]"=w488:refnum<vi>)
                    n324 = property class="DigNum (strict)"(reference=w488) -> (reference out=w484:refnum<vi>, error out=w483:errorcluster, "Value"=w482:i32)  [unwired: 1 in]
                    n325 = Increment(x=w482) -> (x+1=w481:i32)
                    n326 = property class="DigNum (strict)"(reference=w484, error in=w483, "Value"=w481) -> (reference out=w485:refnum<vi>, error out=w486:errorcluster)
                    n327 = Close Reference(reference=w485, error in (no error)=w486) -> ()  [unwired: 1 out]
                  }
                  frame #1 {
                    n328 = Unbundle By Name(w490) -> ("Traction reciepe.SRR INDEX [ TRACTION]"=w495:refnum<vi>)
                    n329 = Unbundle By Name(w490) -> ("Traction reciepe.Traction Size"=w493:refnum<vi>)
                    n330 = property class="DigNum (strict)"(reference=w495) -> (reference out=w497:refnum<vi>, error out=w496:errorcluster, "Value"=w494:i32)  [unwired: 1 in]
                    n331 = property class="DigNum (strict)"(reference=w493) -> (reference out=w491:refnum<vi>, error out=w492:errorcluster, "Value"=w489:i32)  [unwired: 1 in]
                    n332 = Close Reference(reference=w497, error in (no error)=w496) -> ()  [unwired: 1 out]
                    n333 = Close Reference(reference=w491, error in (no error)=w492) -> ()  [unwired: 1 out]
                    n334 = Greater Or Equal?(x=w494, y=w489) -> (x >= y?=w499:bool)
                    n335 = case shown="True" w499 {
                      tunnel: w498 -> [_ w504]
                      frame False {
                      }
                      frame True {
                        n336 = Unbundle By Name(w504) -> ("Traction reciepe.SRR INDEX [ TRACTION]"=w506:refnum<vi>)
                        n337 = Unbundle By Name(w504) -> ("Traction reciepe.Start Index Type"=w514:refnum<vi>)
                        n338 = Unbundle By Name(w504) -> ("Traction reciepe.Start Index Type"=w510:refnum<vi>)
                        n339 = property class="DigNum (strict)"(reference=w510) -> (reference out=w509:refnum<vi>, error out=w511:errorcluster, "Value"=w508:i32)  [unwired: 1 in]
                        n340 = property class="DigNum (strict)"(reference=w506, "Value"=0 ("SRR INDEX [ TRACTION]")) -> (reference out=w505:refnum<vi>, error out=w507:errorcluster)  [unwired: 1 in]
                        n341 = Close Reference(reference=w509, error in (no error)=w511) -> ()  [unwired: 1 out]
                        n342 = Close Reference(reference=w505, error in (no error)=w507) -> ()  [unwired: 1 out]
                        n343 = Increment(x=w508) -> (x+1=w512:i32)
                        n344 = property class="DigNum (strict)"(reference=w514, "Value"=w512) -> (reference out=w513:refnum<vi>, error out=w515:errorcluster)  [unwired: 1 in]
                        n345 = Close Reference(reference=w513, error in (no error)=w515) -> ()  [unwired: 1 out]
                      }
                    }
                    n346 = Select(t=Traction_Receipe_Enum."START" ("Enum - Menu"), s=w499, f=Traction_Receipe_Enum."SRR SET" ("Enum - Menu")) -> (s? t:f=w500:T2)
                  }
                }
                n347 = Unbundle By Name(w464) -> ("Main Screen.Start Test Temp"=w475:refnum<vi>)
                n348 = Unbundle By Name(w464) -> ("Main Screen.STOP"=w478:refnum<vi>)
                n349 = property class="Bool (strict)"(reference=w478) -> (reference out=w480:refnum<vi>, error out=w479:errorcluster, "Value"=w477:bool)  [unwired: 1 in]
                n350 = property class="Bool (strict)"(reference=w475) -> (reference out=w473:refnum<vi>, error out=w474:errorcluster, "Value"=w476:bool)  [unwired: 1 in]
                n351 = Close Reference(reference=w480, error in (no error)=w479) -> ()  [unwired: 1 out]
                n352 = Close Reference(reference=w473, error in (no error)=w474) -> ()  [unwired: 1 out]
                n353 = Equal?(x=w477, y=TRUE) -> (x = y?=w472:bool)
                n354 = Equal?(x=w476, y=FALSE) -> (x = y?=w471:bool)
                n355 = And(x=w472, y=w471) -> (x .and. y?=w468:bool)
                n356 = Select(t=Traction_Receipe_Enum."UNLOAD", s=w468, f=w466) -> (s? t:f=w465:T2)
              }
              frame "STRIBECK" {
                n357 = Unbundle By Name(w517) -> ("Traction reciepe.SRR INDEX [ STRIBECK]"=w534:refnum<vi>)
                n358 = Unbundle By Name(w517) -> ("Traction reciepe.BALL WEAR TRACK"=w544:refnum<vi>)
                n359 = Unbundle By Name(w517) -> ("Traction reciepe.DISC WEARTRACK"=w548:refnum<vi>)
                n360 = Unbundle By Name(w517) -> ("Traction reciepe.Traction Receipe"=w558:refnum<vi>)
                n361 = Unbundle By Name(w517) -> ("Traction reciepe.Start Index Type"=w551:refnum<vi>)
                n362 = Unbundle By Name(w517) -> ("Main Screen.Start Test Temp"=w569:refnum<vi>)
                n363 = Unbundle By Name(w517) -> ("Main Screen.STOP"=w572:refnum<vi>)
                n364 = property class="MCListbox (strict)"(reference=w558) -> (reference out=w556:refnum<vi>, error out=w557:errorcluster, "ItemNames"=w555:string[][])  [unwired: 1 in]
                n365 = property class="DigNum (strict)"(reference=w544) -> (reference out=w542:refnum<vi>, error out=w543:errorcluster, "Value"=w541:dbl)  [unwired: 1 in]
                n366 = property class="DigNum (strict)"(reference=w534) -> (reference out=w536:refnum<vi>, error out=w535:errorcluster, "Value"=w533:i32)  [unwired: 1 in]
                n367 = property class="DigNum (strict)"(reference=w551) -> (reference out=w550:refnum<vi>, error out=w552:errorcluster, "Value"=w549:i32)  [unwired: 1 in]
                n368 = property class="DigNum (strict)"(reference=w548) -> (reference out=w546:refnum<vi>, error out=w547:errorcluster, "Value"=w545:dbl)  [unwired: 1 in]
                n369 = property class="Bool (strict)"(reference=w572) -> (reference out=w574:refnum<vi>, error out=w573:errorcluster, "Value"=w571:bool)  [unwired: 1 in]
                n370 = property class="Bool (strict)"(reference=w569) -> (reference out=w567:refnum<vi>, error out=w568:errorcluster, "Value"=w570:bool)  [unwired: 1 in]
                n371 = Close Reference(reference=w574, error in (no error)=w573) -> ()  [unwired: 1 out]
                n372 = Close Reference(reference=w567, error in (no error)=w568) -> ()  [unwired: 1 out]
                n373 = Close Reference(reference=w542, error in (no error)=w543) -> ()  [unwired: 1 out]
                n374 = Close Reference(reference=w536, error in (no error)=w535) -> ()  [unwired: 1 out]
                n375 = Close Reference(reference=w556, error in (no error)=w557) -> ()  [unwired: 1 out]
                n376 = Close Reference(reference=w550, error in (no error)=w552) -> ()  [unwired: 1 out]
                n377 = Close Reference(reference=w546, error in (no error)=w547) -> ()  [unwired: 1 out]
                n378 = Index Array(array=w555, index (row)=w549) -> (element=w581:string[])  [unwired: 1 in]
                n379 = Equal?(x=w571, y=TRUE) -> (x = y?=w566:bool)
                n380 = Equal?(x=w570, y=FALSE) -> (x = y?=w565:bool)
                n381 = And(x=w566, y=w565) -> (x .and. y?=w562:bool)
                n382 = Index Array(array=w581, index=6) -> (element=w580:string)
                n383 = Index Array(array=w581, index=5) -> (element=w584:string)
                n384 = Unbundle By Name(w517) -> ("Traction reciepe.SET SRR"=w530:refnum<vi>)
                n385 = Select(t=Traction_Receipe_Enum."UNLOAD", s=w562, f=Traction_Receipe_Enum."SPEED SET" ("Enum - Menu")) -> (s? t:f=w559:T2)
                n386 = Fract/Exp String To Number(string=w584) -> (number=w529:dbl)  [unwired: 3 in, 1 out]
                n387 = property class="DigNum (strict)"(reference=w530, "Value"=w529) -> (reference out=w532:refnum<vi>, error out=w531:errorcluster)  [unwired: 1 in]
                n388 = Spreadsheet String To Array(delimiter (Tab)=",", format string="", spreadsheet string=w580, array type (2D Dbl)=string[] []) -> (array=w582:string[])
                n389 = Close Reference(reference=w532, error in (no error)=w531) -> ()  [unwired: 1 out]
                n390 = Unbundle By Name(w517) -> ("Traction reciepe.Stribeck Size"=w526:refnum<vi>)
                n391 = Array Size(array=w582) -> (size(s)=w525:i32)
                n392 = Index Array(array=w582, index=w533) -> (element=w583:string)
                n393 = Divide(x=w529, y=100.0) -> (x/y=w554:dbl)
                n394 = Unbundle By Name(w517) -> ("Traction reciepe.SET entrainment Velocity"=w540:refnum<vi>)
                n395 = Unbundle By Name(w517) -> ("Traction reciepe.DISC SPEED (rpm)"=w522:refnum<vi>)
                n396 = property class="DigNum (strict)"(reference=w526, "Value"=w525) -> (reference out=w528:refnum<vi>, error out=w527:errorcluster)  [unwired: 1 in]
                n397 = Fract/Exp String To Number(string=w583) -> (number=w537:dbl)  [unwired: 3 in, 1 out]
                n398 = property class="DigNum (strict)"(reference=w540, "Value"=w537) -> (reference out=w538:refnum<vi>, error out=w539:errorcluster)  [unwired: 1 in]
                n399 = Close Reference(reference=w528, error in (no error)=w527) -> ()  [unwired: 1 out]
                n400 = call "ENTRAINMENT VELOCITY_SSR TO MM_SEC CONVERSION.vi"("SSR"=w554, "INITIAL Entrainment Speed"=w537) -> ("Disc"=w586:dbl, "Ball"=w585:dbl)  [unwired: 7 in, 1 out]
                n401 = Close Reference(reference=w538, error in (no error)=w539) -> ()  [unwired: 1 out]
                n402 = Unbundle By Name(w517) -> ("Traction reciepe.BALL SPEED (rpm)"=w520:refnum<vi>)
                n403 = call "Rotary mm_s to rpm conversion.vi"("Wear Track Diameter"=w541, "Enter initial Velocity (m/s)  3"=w585) -> ("Initial Speed (RPM) 2"=w516:dbl)  [unwired: 7 in, 2 out]
                n404 = call "Rotary mm_s to rpm conversion.vi"("Wear Track Diameter"=w545, "Enter initial Velocity (m/s)  3"=w586) -> ("Initial Speed (RPM) 2"=w521:dbl)  [unwired: 7 in, 2 out]
                n405 = property class="DigNum (strict)"(reference=w520, "Value"=w516) -> (reference out=w518:refnum<vi>, error out=w519:errorcluster)  [unwired: 1 in]
                n406 = call "Reciepe Ball Speed Write.vi"("Set Speed"=w516, "main ref"=w517) -> ()  [unwired: 9 in, 1 out]
                n407 = property class="DigNum (strict)"(reference=w522, "Value"=w521) -> (reference out=w524:refnum<vi>, error out=w523:errorcluster)  [unwired: 1 in]
                n408 = call "Reciepe Disc Speed Write.vi"("Set Speed"=w521, "main ref"=w517) -> ()  [unwired: 9 in, 1 out]
                n409 = Close Reference(reference=w518, error in (no error)=w519) -> ()  [unwired: 1 out]
                n410 = Close Reference(reference=w524, error in (no error)=w523) -> ()  [unwired: 1 out]
              }
              frame "SPEED SET" {
                w604 = TRUE ("PAUSE")
                n411 = Unbundle By Name(w589) -> ("Main Screen.Start Test Temp"=w598:refnum<vi>)
                n412 = Unbundle By Name(w589) -> ("Main Screen.STOP"=w601:refnum<vi>)
                n413 = property class="Bool (strict)"(reference=w601) -> (reference out=w603:refnum<vi>, error out=w602:errorcluster, "Value"=w600:bool)  [unwired: 1 in]
                n414 = property class="Bool (strict)"(reference=w598) -> (reference out=w596:refnum<vi>, error out=w597:errorcluster, "Value"=w599:bool)  [unwired: 1 in]
                n415 = Close Reference(reference=w603, error in (no error)=w602) -> ()  [unwired: 1 out]
                n416 = Close Reference(reference=w596, error in (no error)=w597) -> ()  [unwired: 1 out]
                n417 = Equal?(x=w600, y=TRUE) -> (x = y?=w595:bool)
                n418 = Equal?(x=w599, y=FALSE) -> (x = y?=w594:bool)
                n419 = And(x=w595, y=w594) -> (x .and. y?=w591:bool)
                n420 = Select(t=Traction_Receipe_Enum."UNLOAD", s=w591, f=Traction_Receipe_Enum."SPEED WAIT" ("Enum - Menu")) -> (s? t:f=w587:T2)
                n421 = call "ELAPSED TIMER VI FOR MM_SEC TRACTION.vi"("RESET"=w604, "PAUSE"=w604) -> ()  [unwired: 7 in, 3 out]
              }
              frame "SPEED WAIT" {
                w637 = FALSE ("PAUSE")
                n422 = Unbundle By Name(w606) -> ("Traction reciepe.Traction Receipe"=w617:refnum<vi>)
                n423 = Unbundle By Name(w606) -> ("Traction reciepe.Start Index Type"=w612:refnum<vi>)
                n424 = Unbundle By Name(w606) -> ("Traction reciepe.ELAPSED TIMER"=w609:refnum<vi>)
                n425 = Unbundle By Name(w606) -> ("Main Screen.Start Test Temp"=w628:refnum<vi>)
                n426 = Unbundle By Name(w606) -> ("Main Screen.STOP"=w631:refnum<vi>)
                n427 = property class="MCListbox (strict)"(reference=w617) -> (reference out=w615:refnum<vi>, error out=w616:errorcluster, "ItemNames"=w614:string[][])  [unwired: 1 in]
                n428 = property class="DigNum (strict)"(reference=w612) -> (reference out=w611:refnum<vi>, error out=w613:errorcluster, "Value"=w610:i32)  [unwired: 1 in]
                n429 = property class="Bool (strict)"(reference=w631) -> (reference out=w633:refnum<vi>, error out=w632:errorcluster, "Value"=w630:bool)  [unwired: 1 in]
                n430 = property class="Bool (strict)"(reference=w628) -> (reference out=w626:refnum<vi>, error out=w627:errorcluster, "Value"=w629:bool)  [unwired: 1 in]
                n431 = Close Reference(reference=w633, error in (no error)=w632) -> ()  [unwired: 1 out]
                n432 = Close Reference(reference=w626, error in (no error)=w627) -> ()  [unwired: 1 out]
                n433 = Close Reference(reference=w615, error in (no error)=w616) -> ()  [unwired: 1 out]
                n434 = Close Reference(reference=w611, error in (no error)=w613) -> ()  [unwired: 1 out]
                n435 = Index Array(array=w614, index (row)=w610) -> (element=w641:string[])  [unwired: 1 in]
                n436 = Equal?(x=w630, y=TRUE) -> (x = y?=w625:bool)
                n437 = Equal?(x=w629, y=FALSE) -> (x = y?=w624:bool)
                n438 = And(x=w625, y=w624) -> (x .and. y?=w621:bool)
                n439 = Index Array(array=w641, index=7) -> (element=w640:string)
                n440 = Fract/Exp String To Number(string=w640) -> (number=w638:dbl)  [unwired: 3 in, 1 out]
                n441 = call "ELAPSED TIMER VI FOR MM_SEC TRACTION.vi"("TARGET"=w638, "RESET"=w637, "PAUSE"=w637) -> ("ELAPSED INDICATION"=w634:bool, "ELAPSED TIMER"=w605:dbl)  [unwired: 6 in, 1 out]
                n442 = property class="DigNum (strict)"(reference=w609, "Value"=w605) -> (reference out=w607:refnum<vi>, error out=w608:errorcluster)  [unwired: 1 in]
                n443 = Select(t=Traction_Receipe_Enum."SPEED INCREMENT" ("Enum - Menu"), s=w634, f=Traction_Receipe_Enum."SPEED WAIT") -> (s? t:f=w619:T2)
                n444 = Close Reference(reference=w607, error in (no error)=w608) -> ()  [unwired: 1 out]
                n445 = Select(t=Traction_Receipe_Enum."UNLOAD", s=w621, f=w619) -> (s? t:f=w618:T2)
              }
              frame "SPEED INCREMENT" {
                n446 = flat-sequence {
                  tunnel: w642 -> [w665]
                  tunnel: [w684] -> w664
                  tunnel: w642 -> [w674]
                  tunnel: [w674] -> w643
                  tunnel: [w712] -> w649
                  tunnel: w664 -> [w711]
                  tunnel: w644 -> [w709]
                  tunnel: w643 -> [w705]
                  frame #0 {
                    n447 = Unbundle By Name(w665) -> ("Traction reciepe.SRR INDEX [ STRIBECK]"=w666:refnum<vi>)
                    n448 = property class="DigNum (strict)"(reference=w666) -> (reference out=w669:refnum<vi>, error out=w670:errorcluster, "Value"=w671:i32)  [unwired: 1 in]
                    n449 = Increment(x=w671) -> (x+1=w672:i32)
                    n450 = property class="DigNum (strict)"(reference=w669, error in=w670, "Value"=w672) -> (reference out=w668:refnum<vi>, error out=w667:errorcluster)
                    n451 = Close Reference(reference=w668, error in (no error)=w667) -> ()  [unwired: 1 out]
                  }
                  frame #1 {
                    n452 = Unbundle By Name(w674) -> ("Traction reciepe.SRR INDEX [ STRIBECK]"=w675:refnum<vi>)
                    n453 = Unbundle By Name(w674) -> ("Traction reciepe.Stribeck Size"=w680:refnum<vi>)
                    n454 = property class="DigNum (strict)"(reference=w680) -> (reference out=w678:refnum<vi>, error out=w679:errorcluster, "Value"=w682:i32)  [unwired: 1 in]
                    n455 = property class="DigNum (strict)"(reference=w675) -> (reference out=w677:refnum<vi>, error out=w676:errorcluster, "Value"=w681:i32)  [unwired: 1 in]
                    n456 = Close Reference(reference=w678, error in (no error)=w679) -> ()  [unwired: 1 out]
                    n457 = Close Reference(reference=w677, error in (no error)=w676) -> ()  [unwired: 1 out]
                    n458 = Greater Or Equal?(x=w681, y=w682) -> (x >= y?=w673:bool)
                    n459 = case shown="True" w673 {
                      tunnel: w674 -> [_ w689]
                      frame False {
                      }
                      frame True {
                        n460 = Unbundle By Name(w689) -> ("Traction reciepe.SRR INDEX [ STRIBECK]"=w690:refnum<vi>)
                        n461 = Unbundle By Name(w689) -> ("Traction reciepe.Start Index Type"=w691:refnum<vi>)
                        n462 = property class="DigNum (strict)"(reference=w691) -> (reference out=w694:refnum<vi>, error out=w695:errorcluster, "Value"=w696:i32)  [unwired: 1 in]
                        n463 = property class="DigNum (strict)"(reference=w690, "Value"=0 ("SRR INDEX [ STRIBECK]")) -> (reference out=w687:refnum<vi>, error out=w688:errorcluster)  [unwired: 1 in]
                        n464 = Increment(x=w696) -> (x+1=w697:i32)
                        n465 = Close Reference(reference=w687, error in (no error)=w688) -> ()  [unwired: 1 out]
                        n466 = property class="DigNum (strict)"(reference=w694, error in=w695, "Value"=w697) -> (reference out=w693:refnum<vi>, error out=w692:errorcluster)
                        n467 = Close Reference(reference=w693, error in (no error)=w692) -> ()  [unwired: 1 out]
                      }
                    }
                    n468 = Select(t=Traction_Receipe_Enum."START" ("Enum - Menu"), s=w673, f=Traction_Receipe_Enum."STRIBECK") -> (s? t:f=w684:T2)
                  }
                  frame #2 {
                    n469 = Unbundle By Name(w705) -> ("Traction reciepe.Start Index Type"=w706:refnum<vi>)
                    n470 = property class="DigNum (strict)"(reference=w706) -> (reference out=w708:refnum<vi>, error out=w707:errorcluster, "Value"=w704:i32)  [unwired: 1 in]
                    n471 = Index Array(array=w709, index (row)=w704) -> (element=w715:string[])  [unwired: 1 in]
                    n472 = Close Reference(reference=w708, error in (no error)=w707) -> ()  [unwired: 1 out]
                    n473 = Index Array(array=w715, index=1) -> (element=w703:string)
                    n474 = Equal?(x=w703, y="\"TRACTION\"") -> (x = y?=w700:bool)
                    n475 = call <vilib>:"Trim Whitespace.vi"("string"=w703) -> ("trimmed string"=w701:string)  [unwired: 1 in]
                    n476 = Equal?(x=w701, y="") -> (x = y?=w699:bool)
                    n477 = Or(x=w700, y=w699) -> (x .or. y?=w698:bool)
                    n478 = Select(t=Traction_Receipe_Enum."UNLOAD", s=w698, f=w711) -> (s? t:f=w712:T2)
                  }
                }
                n479 = Unbundle By Name(w642) -> ("Traction reciepe.Traction Receipe"=w647:refnum<vi>)
                n480 = Unbundle By Name(w642) -> ("Main Screen.Start Test Temp"=w658:refnum<vi>)
                n481 = Unbundle By Name(w642) -> ("Main Screen.STOP"=w661:refnum<vi>)
                n482 = property class="MCListbox (strict)"(reference=w647) -> (reference out=w645:refnum<vi>, error out=w646:errorcluster, "ItemNames"=w644:string[][])  [unwired: 1 in]
                n483 = property class="Bool (strict)"(reference=w661) -> (reference out=w663:refnum<vi>, error out=w662:errorcluster, "Value"=w660:bool)  [unwired: 1 in]
                n484 = property class="Bool (strict)"(reference=w658) -> (reference out=w656:refnum<vi>, error out=w657:errorcluster, "Value"=w659:bool)  [unwired: 1 in]
                n485 = Close Reference(reference=w663, error in (no error)=w662) -> ()  [unwired: 1 out]
                n486 = Close Reference(reference=w656, error in (no error)=w657) -> ()  [unwired: 1 out]
                n487 = Close Reference(reference=w645, error in (no error)=w646) -> ()  [unwired: 1 out]
                n488 = Equal?(x=w660, y=TRUE) -> (x = y?=w655:bool)
                n489 = Equal?(x=w659, y=FALSE) -> (x = y?=w654:bool)
                n490 = And(x=w655, y=w654) -> (x .and. y?=w651:bool)
                n491 = Select(t=Traction_Receipe_Enum."UNLOAD", s=w651, f=w649) -> (s? t:f=w648:T2)
              }
              frame "UNLOAD" {
                (unwired) FALSE ("Value")
                n492 = call "Test Stop Traction.vi"("Data Cluster"=w718) -> ()  [unwired: 10 in, 1 out]
                n493 = Unbundle By Name(w718) -> ("Traction reciepe.Start Index Type"=w719:refnum<vi>)
                n494 = Unbundle By Name(w718) -> ("Main Screen.Start Test Temp"=w748:refnum<vi>)
                n495 = Unbundle By Name(w718) -> ("Traction reciepe.Test Array Size"=w723:refnum<vi>)
                n496 = Unbundle By Name(w718) -> ("Main Screen.Load En"=w734:refnum<vi>)
                n497 = Unbundle By Name(w718) -> ("Main Screen.STOP"=w751:refnum<vi>)
                n498 = Unbundle By Name(w718) -> ("Main Screen.zNL 2"=w729:refnum<vi>)
                n499 = property on="Property Node" class="DigNum (strict)"(reference=w719) -> (reference out=w717:refnum<vi>, error out=w720:errorcluster, "Value"=w716:i32)  [unwired: 1 in]
                n500 = property class="DigNum (strict)"(reference=w723) -> (reference out=w722:refnum<vi>, error out=w724:errorcluster, "Value"=w721:i32)  [unwired: 1 in]
                n501 = property on="Property Node" class="Bool (strict)"(reference=w734, "Value"=FALSE) -> (reference out=w732:refnum<vi>, error out=w733:errorcluster)  [unwired: 1 in]
                n502 = property class="Bool (strict)"(reference=w751) -> (reference out=w753:refnum<vi>, error out=w752:errorcluster, "Value"=w750:bool)  [unwired: 1 in]
                n503 = property class="Bool (strict)"(reference=w748) -> (reference out=w746:refnum<vi>, error out=w747:errorcluster, "Value"=w749:bool)  [unwired: 1 in]
                n504 = Close Reference(reference=w753, error in (no error)=w752) -> ()  [unwired: 1 out]
                n505 = Close Reference(reference=w746, error in (no error)=w747) -> ()  [unwired: 1 out]
                n506 = Close Reference(reference=w717, error in (no error)=w720) -> ()  [unwired: 1 out]
                n507 = Close Reference(reference=w722, error in (no error)=w724) -> ()  [unwired: 1 out]
                n508 = Close Reference(reference=w732, error in (no error)=w733) -> (error out=w728:errorcluster)
                n509 = Decrement(x=w721) -> (x-1=w754:i32)
                n510 = Equal?(x=w750, y=TRUE) -> (x = y?=w745:bool)
                n511 = Equal?(x=w749, y=FALSE) -> (x = y?=w744:bool)
                n512 = property on="Property Node" class="Bool (strict)"(reference=w729, error in=w728, "DisabledEnum"=T3."Enabled" ("Disabled")) -> (reference out=w731:refnum<vi>, error out=w730:errorcluster)
                n513 = Greater Or Equal?(x=w716, y=w754) -> (x >= y?=w757:bool)
                n514 = And(x=w745, y=w744) -> (x .and. y?=w741:bool)
                n515 = Select(t=Traction_Receipe_Enum."CLOSE" ("Enum - Menu"), s=w757, f=Traction_Receipe_Enum."START" ("Enum - Menu")) -> (s? t:f=w739:T2)
                n516 = Close Reference(reference=w731, error in (no error)=w730) -> (error out=w725:errorcluster)
                n517 = Select(t=Traction_Receipe_Enum."CLOSE", s=w741, f=w739) -> (s? t:f=w738:T2)
                n518 = call "Reciepe Ball Speed Write.vi"("error in (no error)"=w725, "Set Speed"=0.0, "main ref"=w718) -> ("error out"=w735:errorcluster)  [unwired: 8 in]
                n519 = call "Reciepe Disc Speed Write.vi"("error in (no error)"=w735, "Set Speed"=0.0, "main ref"=w718) -> ()  [unwired: 8 in, 1 out]
              }
              frame "CLOSE" {
                w759 = 0 ("Start Index")
                n520 = call "Test Stop.vi"("Data Cluster"=w758) -> ()  [unwired: 10 in, 1 out]
                n521 = Unbundle By Name(w758) -> ("Traction reciepe.SRR INDEX [ TRACTION]"=w763:refnum<vi>)
                n522 = Unbundle By Name(w758) -> ("Traction reciepe.SRR INDEX [ STRIBECK]"=w760:refnum<vi>)
                n523 = Unbundle By Name(w758) -> ("Traction reciepe.Start Index Type"=w767:refnum<vi>)
                n524 = property class="DigNum (strict)"(reference=w767, "Value"=w759) -> (reference out=w766:refnum<vi>, error out=w768:errorcluster)  [unwired: 1 in]
                n525 = property class="DigNum (strict)"(reference=w763, "Value"=w759) -> (reference out=w765:refnum<vi>, error out=w764:errorcluster)  [unwired: 1 in]
                n526 = property class="DigNum (strict)"(reference=w760, "Value"=w759) -> (reference out=w762:refnum<vi>, error out=w761:errorcluster)  [unwired: 1 in]
                n527 = Close Reference(reference=w766, error in (no error)=w768) -> ()  [unwired: 1 out]
                n528 = Close Reference(reference=w765, error in (no error)=w764) -> ()  [unwired: 1 out]
                n529 = Close Reference(reference=w762, error in (no error)=w761) -> ()  [unwired: 1 out]
              }
            }
            n530 = Wait (ms)(milliseconds to wait=u32 300) -> ()  [unwired: 1 out]
            n531 = property class="Enum (strict)"(reference=w22, "Value"=w19) -> (reference out=w20:refnum<vi>, error out=w23:errorcluster)  [unwired: 1 in]
            n532 = Close Reference(reference=w20, error in (no error)=w23) -> ()  [unwired: 1 out]
          }
        }
      }
    }
    frame Error {
    }
  }
